vi "Spectrometer.vi"(0 "Function":T14, 3 "Labram HR Notifications":T13, 5 "Laser Settings":T5={"Laser Wavelength"=enum."633 nm", "Neutral Density Filter"=enum."1%"}, 7 "Spectrometer Settings":T2={"Confocal Hole Size (µm)"=150.0, "Grating"=1, "Detector"=enum."InGaAs Array"} {"Grating" items=["1800 l/mm", "150 l/mm"]}, 9 "Acquisition Settings":T1={"Acquisition Mode"=enum."Single Window", "Spectal Position (nm)"=480.0, "From (nm)"=632.0, "To (nm)"=1000.0, "Integration Time (s)"=3.0, "Number of Accumulations"=3, "AutoScanning"=FALSE, "Spike Removal"=FALSE}, 11 "error in":errorcluster, 12 "Optical Spectrum":enum32{"Energy", "Wavelength", "Raman Shift"}(tab), 13 "Path":path, 14 "LabramHR References":T8) -> (4 "Spectrum":T10, 6 "Laser Settings Out":T5={"Laser Wavelength"=enum."633 nm", "Neutral Density Filter"=enum."1%"}, 8 "Spectrometer Settings Out":T2={"Confocal Hole Size (µm)"=150.0, "Grating"=1, "Detector"=enum."InGaAs Array"} {"Grating" items=["1800 l/mm", "150 l/mm"]}, 10 "Acquisition Settings Out":T1={"Acquisition Mode"=enum."Single Window", "Spectal Position (nm)"=480.0, "From (nm)"=632.0, "To (nm)"=1000.0, "Integration Time (s)"=3.0, "Number of Accumulations"=3, "AutoScanning"=FALSE, "Spike Removal"=FALSE}, 15 "error out":errorcluster)   [LabVIEW 2014]
uses:
  Spectrometer Function.ctl
  Spectrometer Notifiers.ctl
  support/Instrument Status.ctl
  Laser Settings.ctl
  Laser.ctl
  Filter.ctl
  Grating Detector Settings.ctl
  Grating.ctl
  Detector.ctl
  Acquisition Settings.ctl
  Spectral Data.ctl
  Spectrometer Refnum.ctl
  Measurements/Plot Data/Optical Spectrum Plot Refnum.ctl
  MoveMotor Motor Name.ctl
  support/Instrument Status State.ctl
  Spectrometer Config.ctl
  Acquire Mode.ctl
  Acquire Shutter Mode.ctl
  Acquire Data Handling.ctl
panel:
  out "Detector Temperature":dbl
  out "Optical Spectrum vs Energy":cluster{"data":dbl[], "data":dbl[]}(graph)
  out "Optical Spectrum vs Wavelength":cluster{"data":dbl[], "data":dbl[]}(graph)
  out "Optical Spectrum vs Raman Shift":cluster{"data":dbl[], "data":dbl[]}(graph)
  out "Motor ID":T11={"Laser"=-1, "Hole"=-1, "Filter"=-1, "Grating"=-1, "Spectro"=-1, "Detector"=-1}
  out "Instrument Status":T12
  # "LICENSED MATERIALS – PROPERTY OF IBM\nCopyright IBM Corp. 2016,\nALL RIGHTS RESERVED"
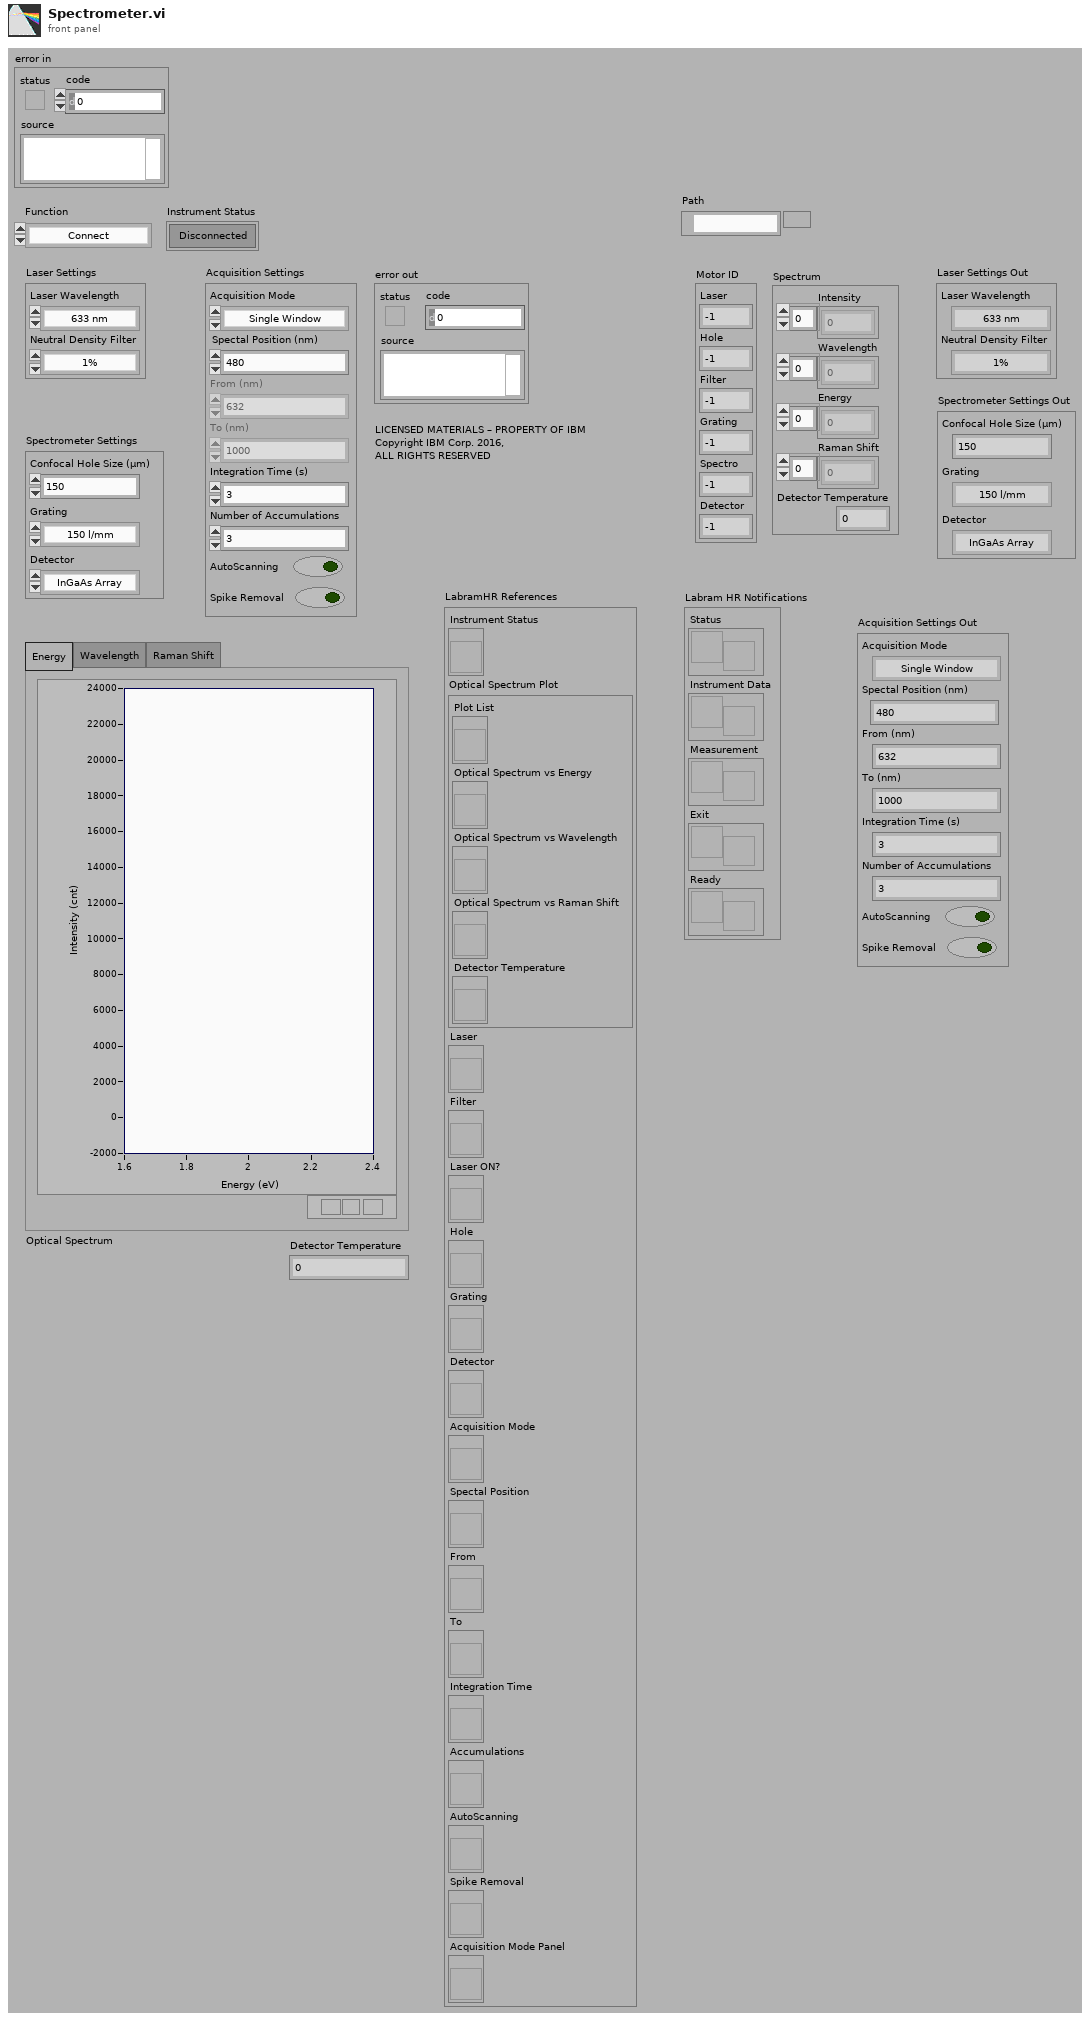
[diagram p1: front panel]
types:
  T1 = typedef "Acquisition Settings.ctl" = cluster{"Acquisition Mode":enum16{"Single Window", "Multi-Window"}, "Spectal Position (nm)":dbl, "From (nm)":dbl, "To (nm)":dbl, "Integration Time (s)":dbl, "Number of Accumulations":i32, "AutoScanning":bool, "Spike Removal":bool}
  T2 = typedef "Grating Detector Settings.ctl" = cluster{"Confocal Hole Size (µm)":dbl, "Grating":T3, "Detector":T4}
  T3 = typedef "Grating.ctl" = u16
  T4 = typedef "Detector.ctl" = enum16{"InGaAs Array", "Silicon CCD"}
  T5 = typedef "Laser Settings.ctl" = cluster{"Laser Wavelength":T6, "Neutral Density Filter":T7}
  T6 = typedef "Laser.ctl" = enum16{"633 nm", "784 nm", "532 nm", "365 nm"}
  T7 = typedef "Filter.ctl" = enum16{"100%", "50%", "25%", "10%", "1%", "0.1%", "0.01%"}
  T8 = typedef "Spectrometer Refnum.ctl" = cluster{"Instrument Status":refnum<vi>, "Optical Spectrum Plot":T9, "Laser":refnum<vi>, "Filter":refnum<vi>, "Laser ON?":refnum<vi>, "Hole":refnum<vi>, "Grating":refnum<vi>, "Detector":refnum<vi>, "Acquisition Mode":refnum<vi>, "Spectal Position":refnum<vi>, "From":refnum<vi>, "To":refnum<vi>, "Integration Time":refnum<vi>, "Accumulations":refnum<vi>, "AutoScanning":refnum<vi>, "Spike Removal":refnum<vi>, "Acquisition Mode Panel":refnum<vi>}
  T9 = typedef "Optical Spectrum Plot Refnum.ctl" = cluster{"Plot List":refnum<vi>, "Optical Spectrum vs Energy":refnum<vi>, "Optical Spectrum vs Wavelength":refnum<vi>, "Optical Spectrum vs Raman Shift":refnum<vi>, "Detector Temperature":refnum<vi>}
  T10 = typedef "Spectral Data.ctl" = cluster{"Intensity":dbl[], "Wavelength":dbl[], "Energy":dbl[], "Raman Shift":dbl[], "Detector Temperature":dbl}
  T11 = cluster{"Laser":i32, "Hole":i32, "Filter":i32, "Grating":i32, "Spectro":i32, "Detector":i32}
  T12 = typedef "Instrument Status.ctl" = bool
  T13 = typedef "Spectrometer Notifiers.ctl" = cluster{"Status":refnum<notifier>, "Instrument Data":refnum<notifier>, "Measurement":refnum<notifier>, "Exit":refnum<notifier>, "Ready":refnum<notifier>}
  T14 = typedef "Spectrometer Function.ctl" = enum16{"Connect", "Complete Configuration", "Get Status", "Load Configuration", "Save Configuration", "Acquire Spectrum", "Read File", "Set Laser", "Set Filter", "Set Hole", "Set Grating", "Set Grating Position", "Set Detector", "Set Acquisition Mode", "Update Refnums", "Disconnect"}
  T15 = enum16{"Generic Data", "Spectrum", "Spectral Profile Image", "Map", "Video", "First Data", "Next Data"}
  T16 = typedef "Instrument Status State.ctl" = enum16{"Unknown", "Idle", "Standby", "Configuring", "Measuring", "Moving", "Disconnected"}
  T17 = typedef "MoveMotor Motor Name.ctl" = enum16{"Spectro", "Premono", "Grating", "Slit", "Hole", "X", "Y", "XT", "YT", "XL", "YL", "Z", "Laser", "Filter", "Objective", "Detector", "Detector Temperature"}
  T18 = typedef "Spectrometer Config.ctl" = cluster{"Laser Settings":T5, "Spectrometer Settings":T2, "Acquisition Settings":T1, "Path":path}
  T19 = enum8{"Enabled", "Disabled", "Disabled and Grayed Out"}
  T20 = cluster{"Optical Spectrum vs Energy":cluster{"Intensity":dbl[], "Energy":dbl[]}, "Optical Spectrum vs Wavelength":cluster{"Intensity":dbl[], "Wavelength":dbl[]}, "Optical Spectrum vs Raman Shift":cluster{"Intensity":dbl[], "Raman Shift":dbl[]}}
  T21 = typedef "Acquire Mode.ctl" = u16
  T22 = typedef "Acquire Shutter Mode.ctl" = u16
  T23 = typedef "Acquire Data Handling.ctl" = u16
  T24 = enum8{"Enabled", "Disabled", "Disabled and Grayed Out"}[]
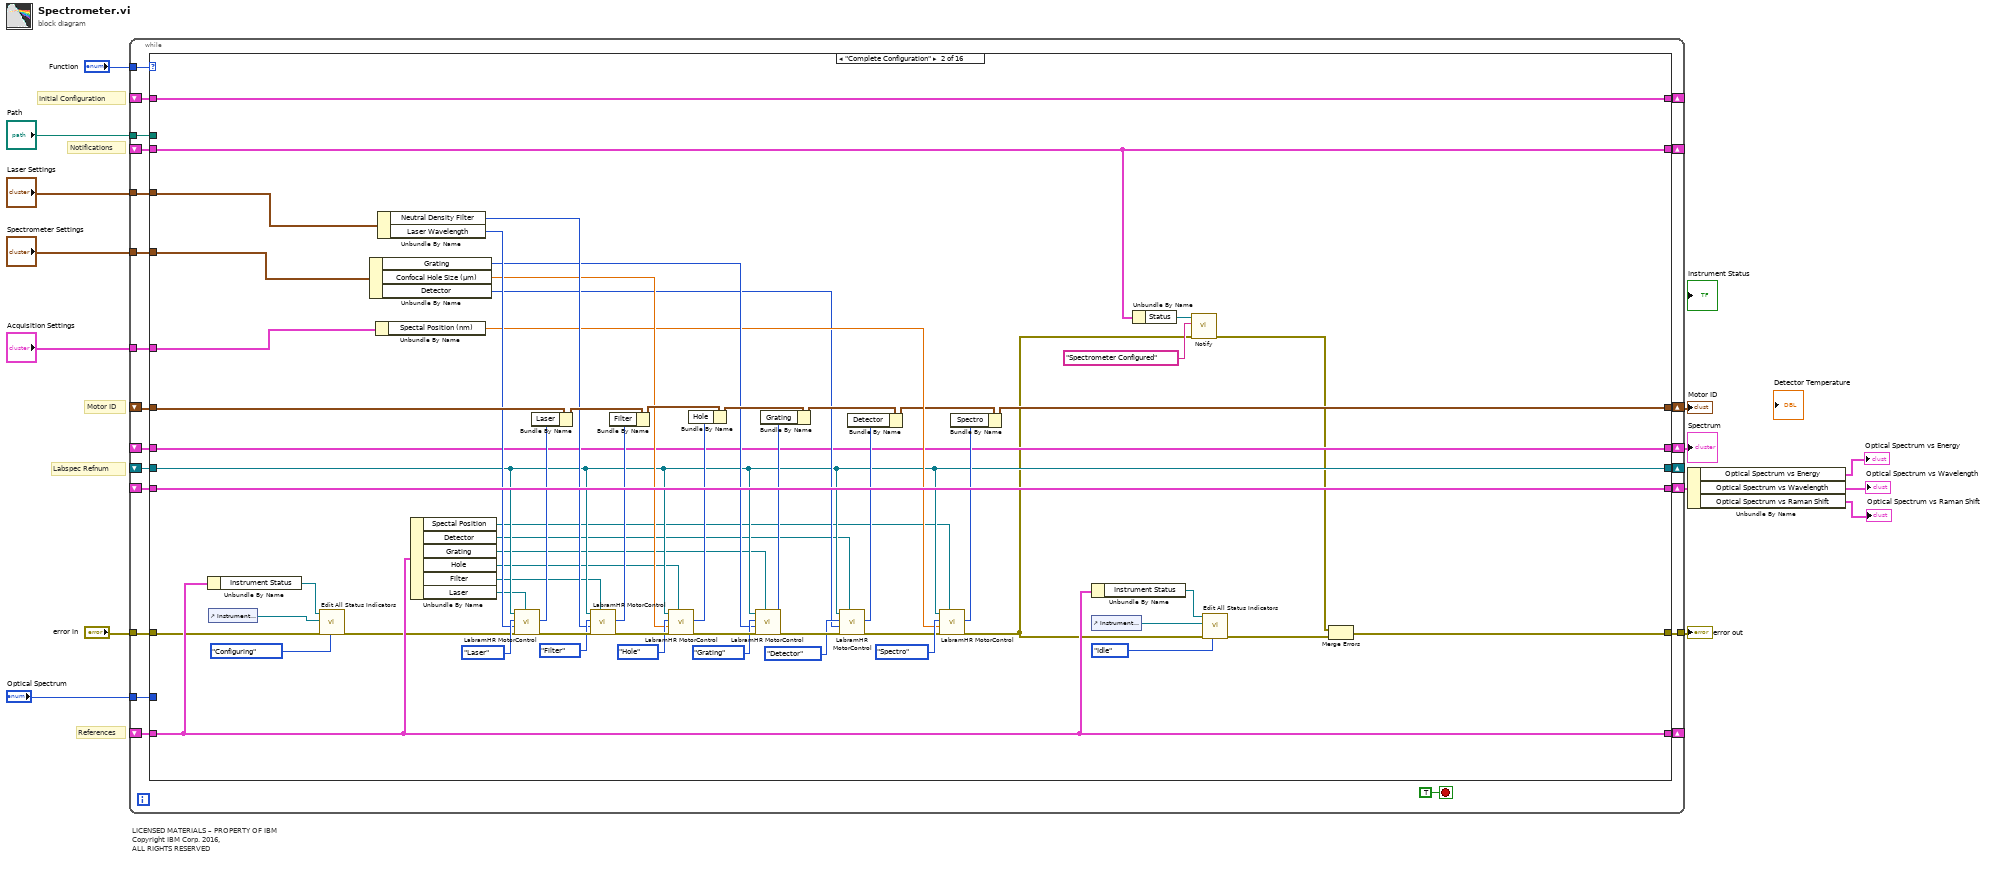
[diagram p0: block diagram]
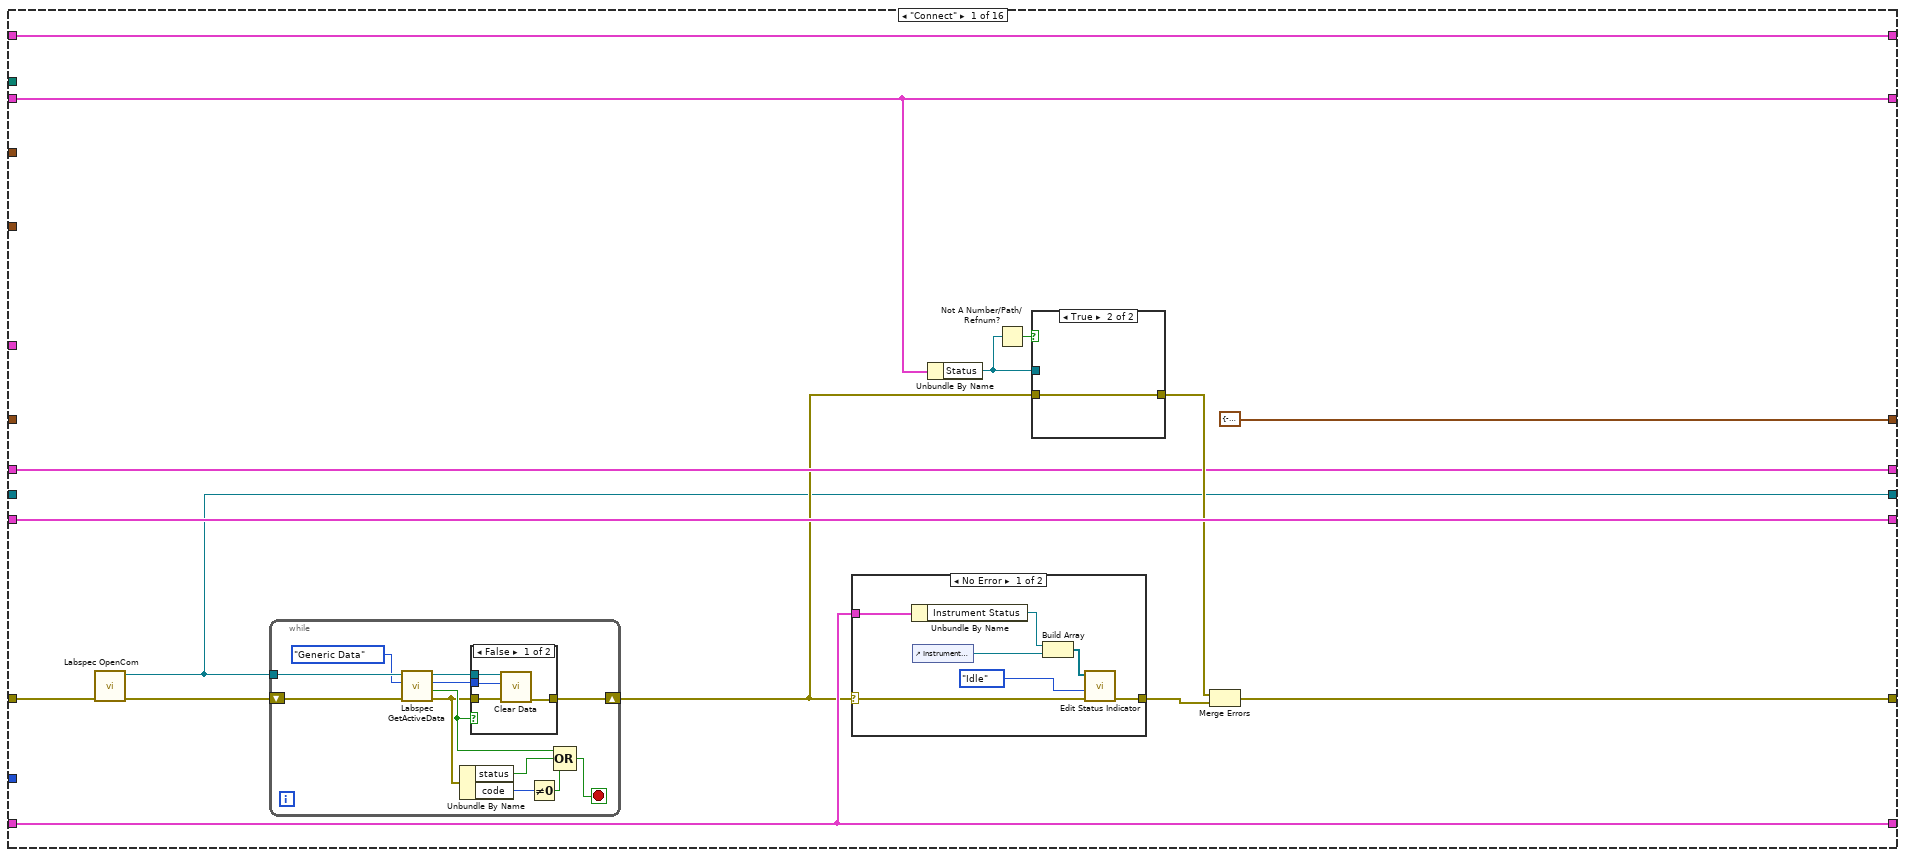
[diagram p2: hidden frame]
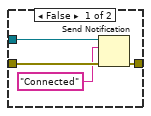
[diagram p4: hidden frame]
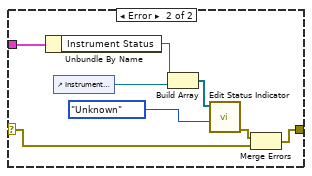
[diagram p5: hidden frame]
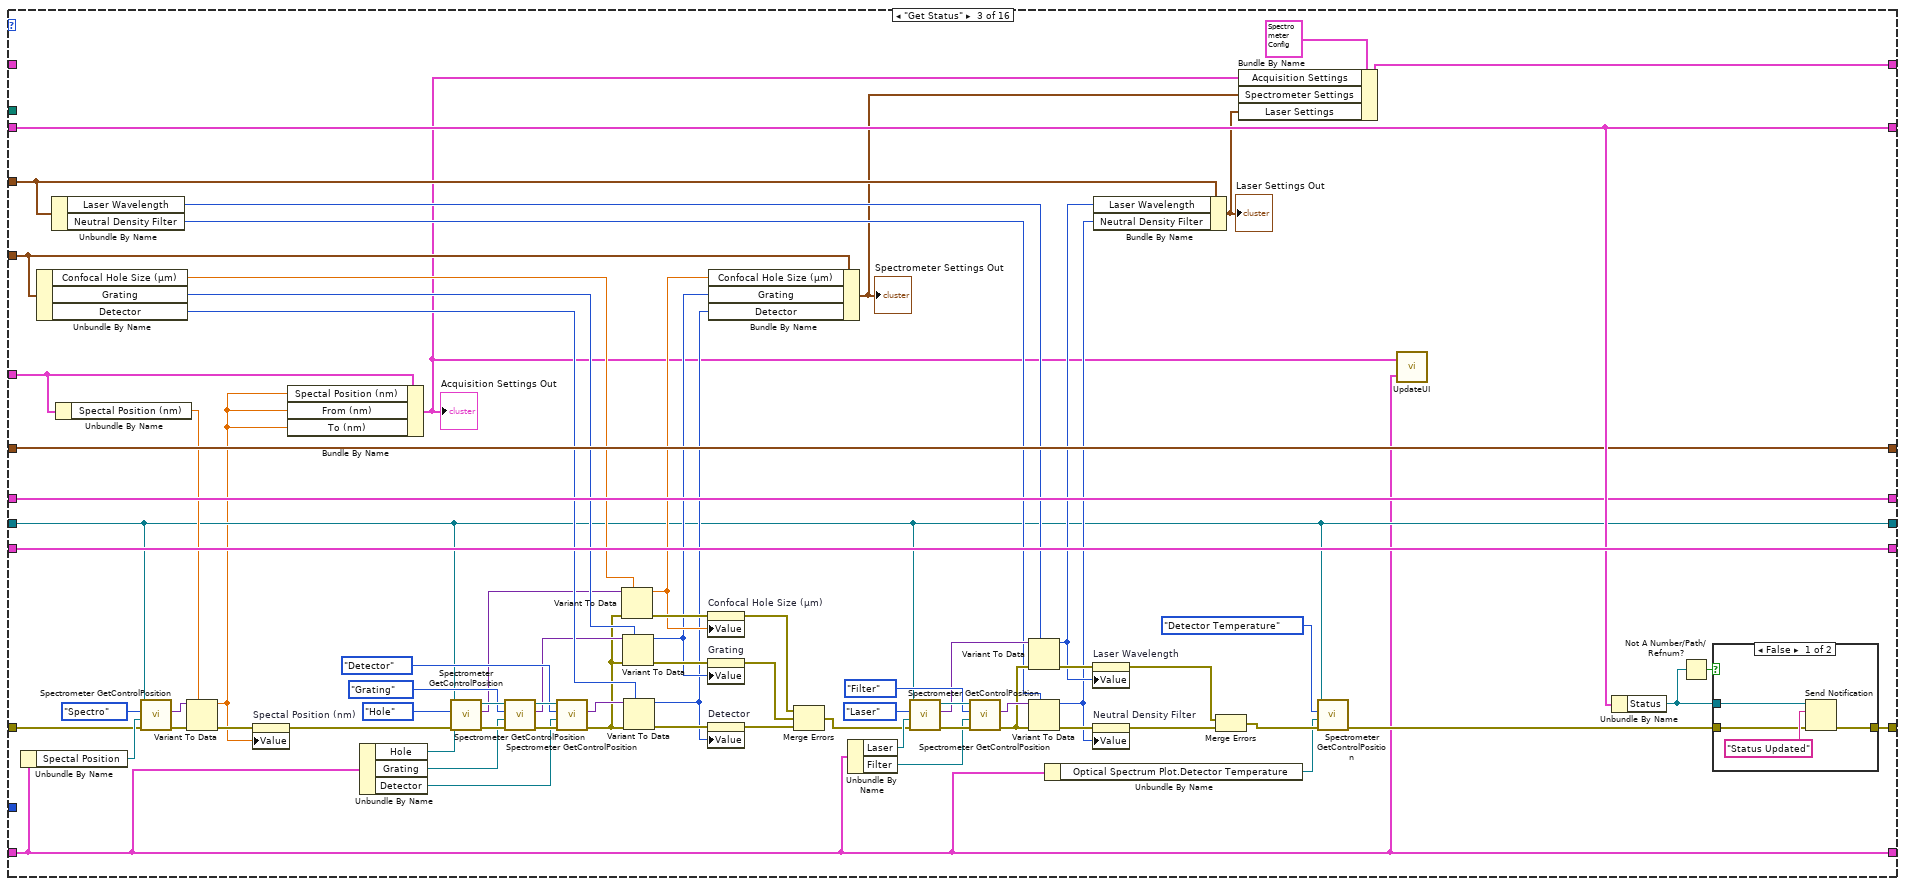
[diagram p6: hidden frame]
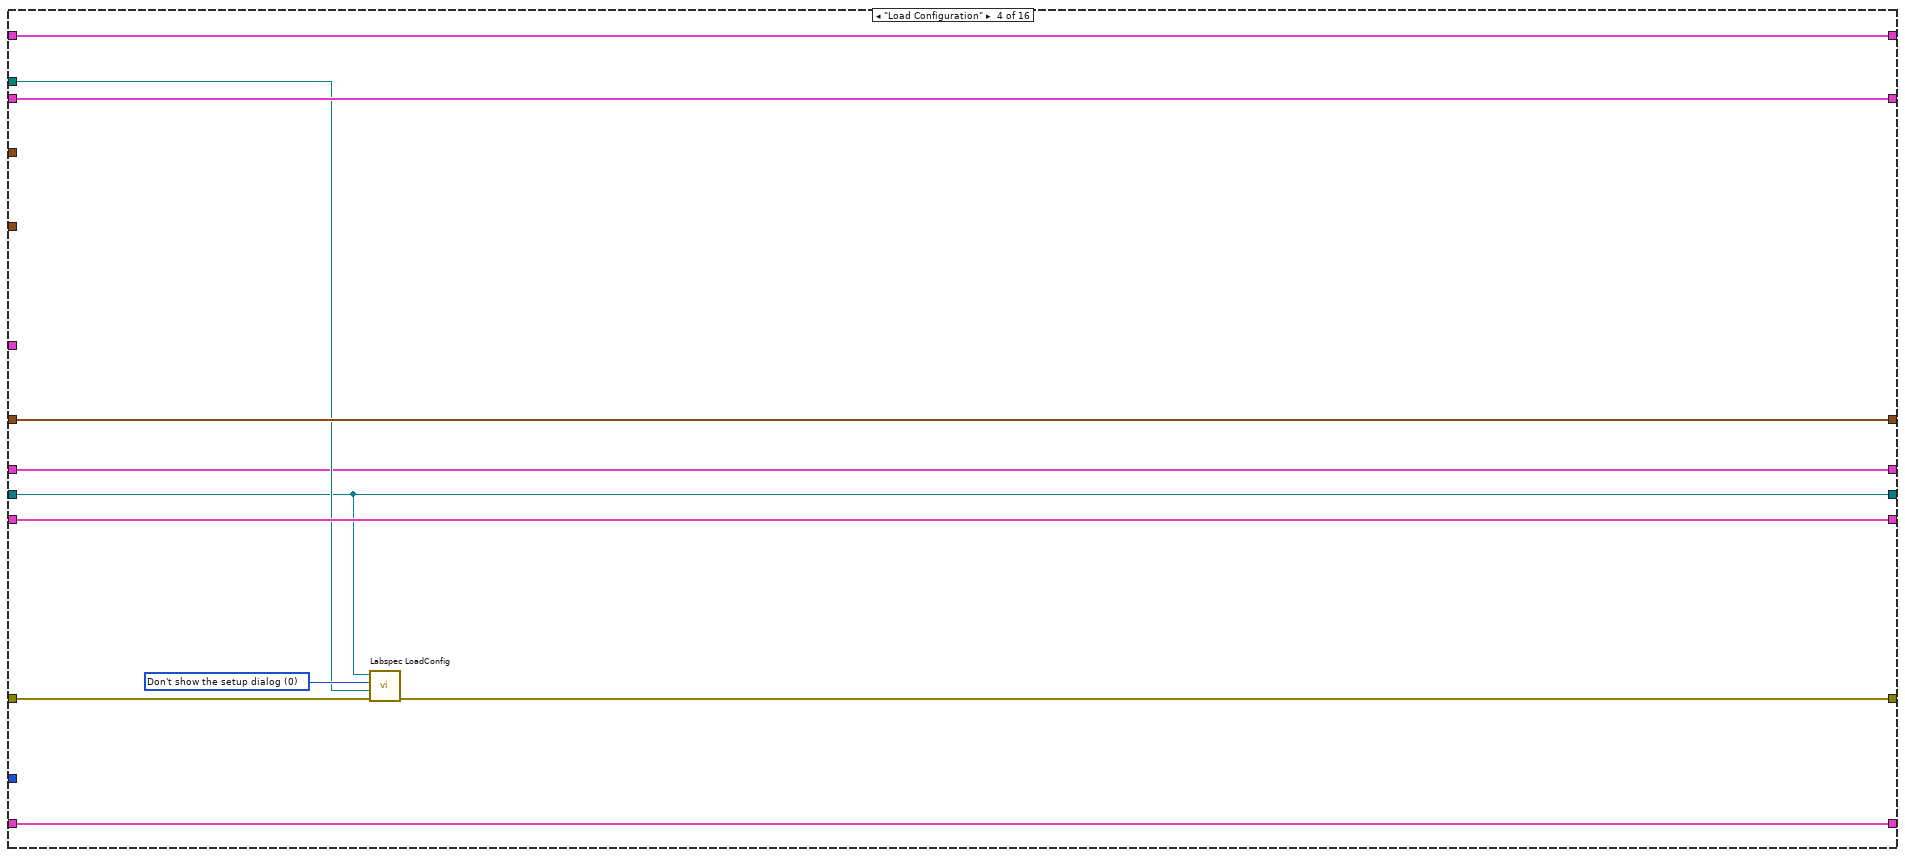
[diagram p8: hidden frame]
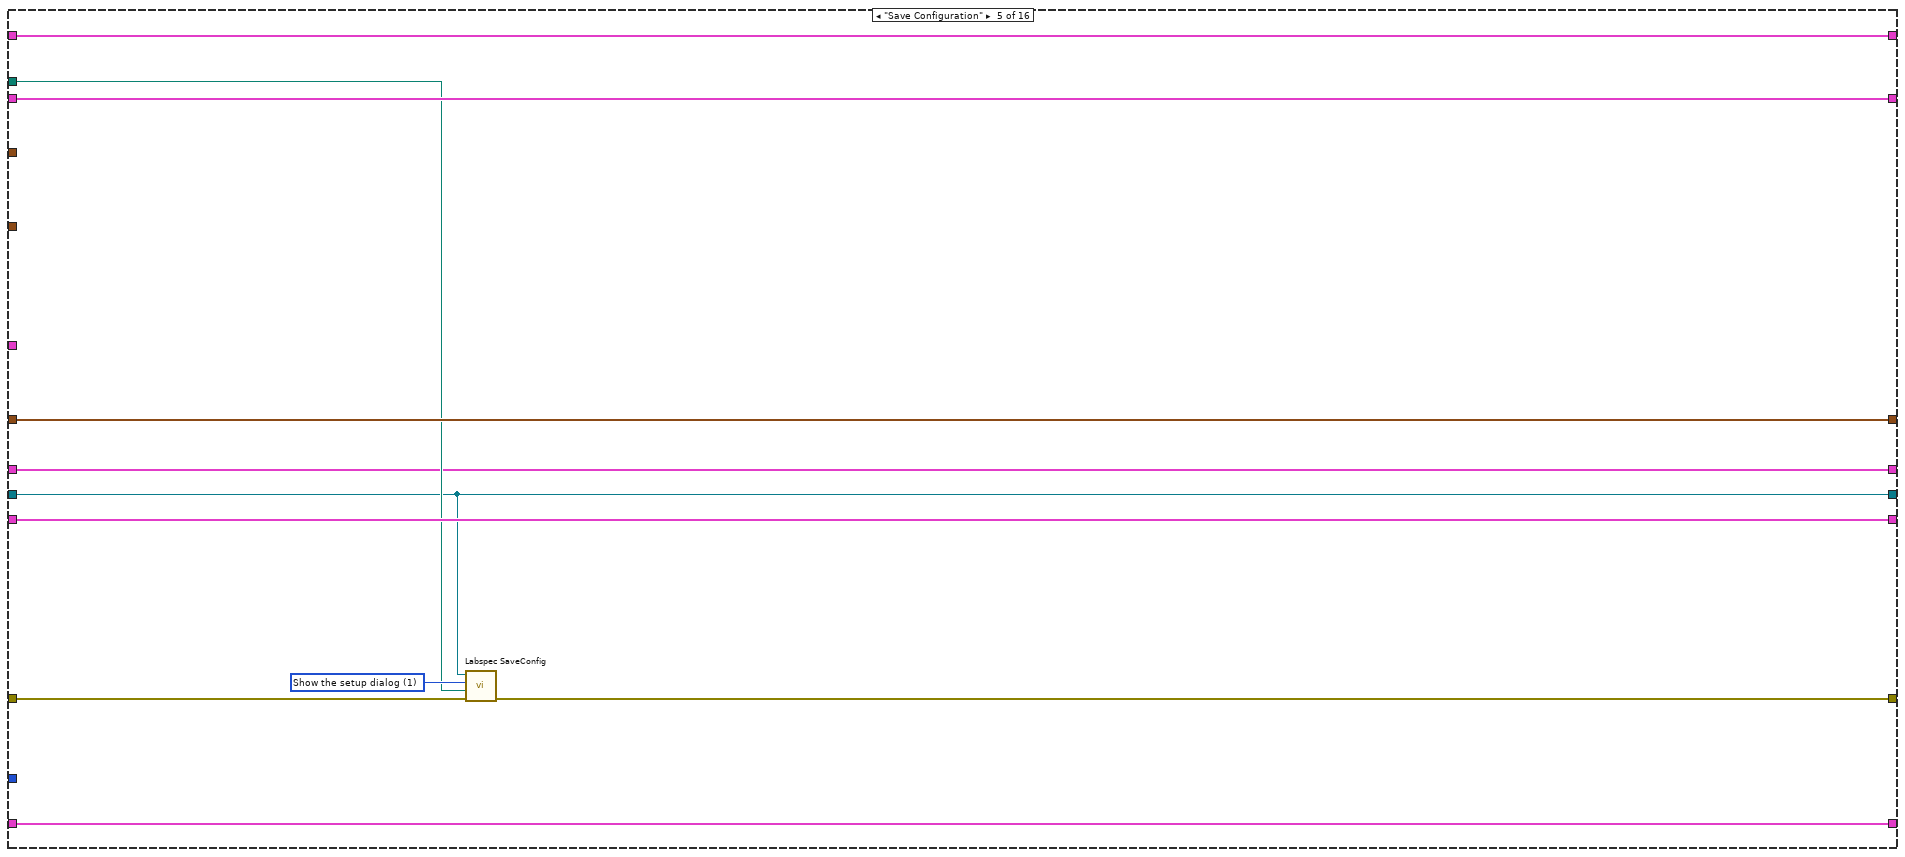
[diagram p9: hidden frame]
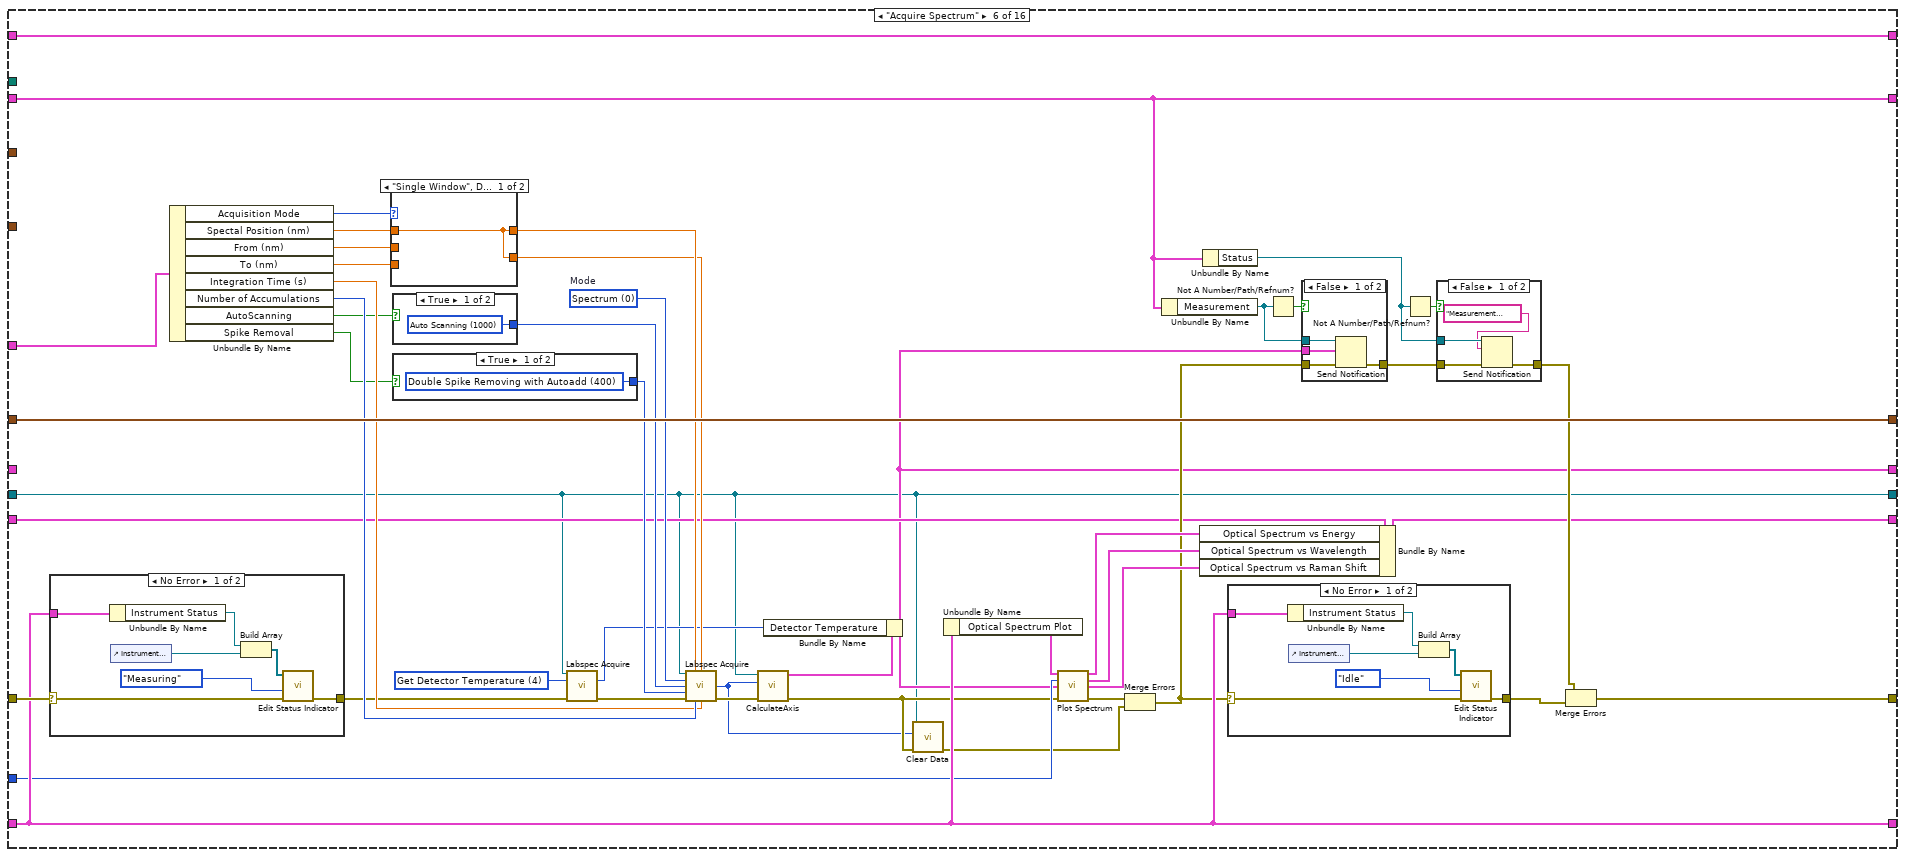
[diagram p10: hidden frame]
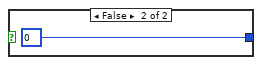
[diagram p13: hidden frame]
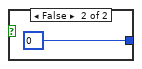
[diagram p14: hidden frame]
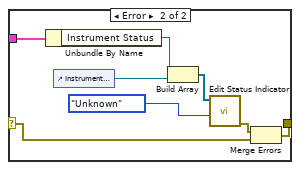
[diagram p15: hidden frame]
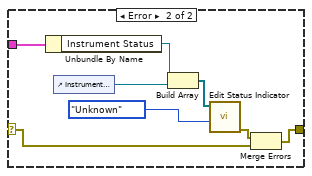
[diagram p16: hidden frame]
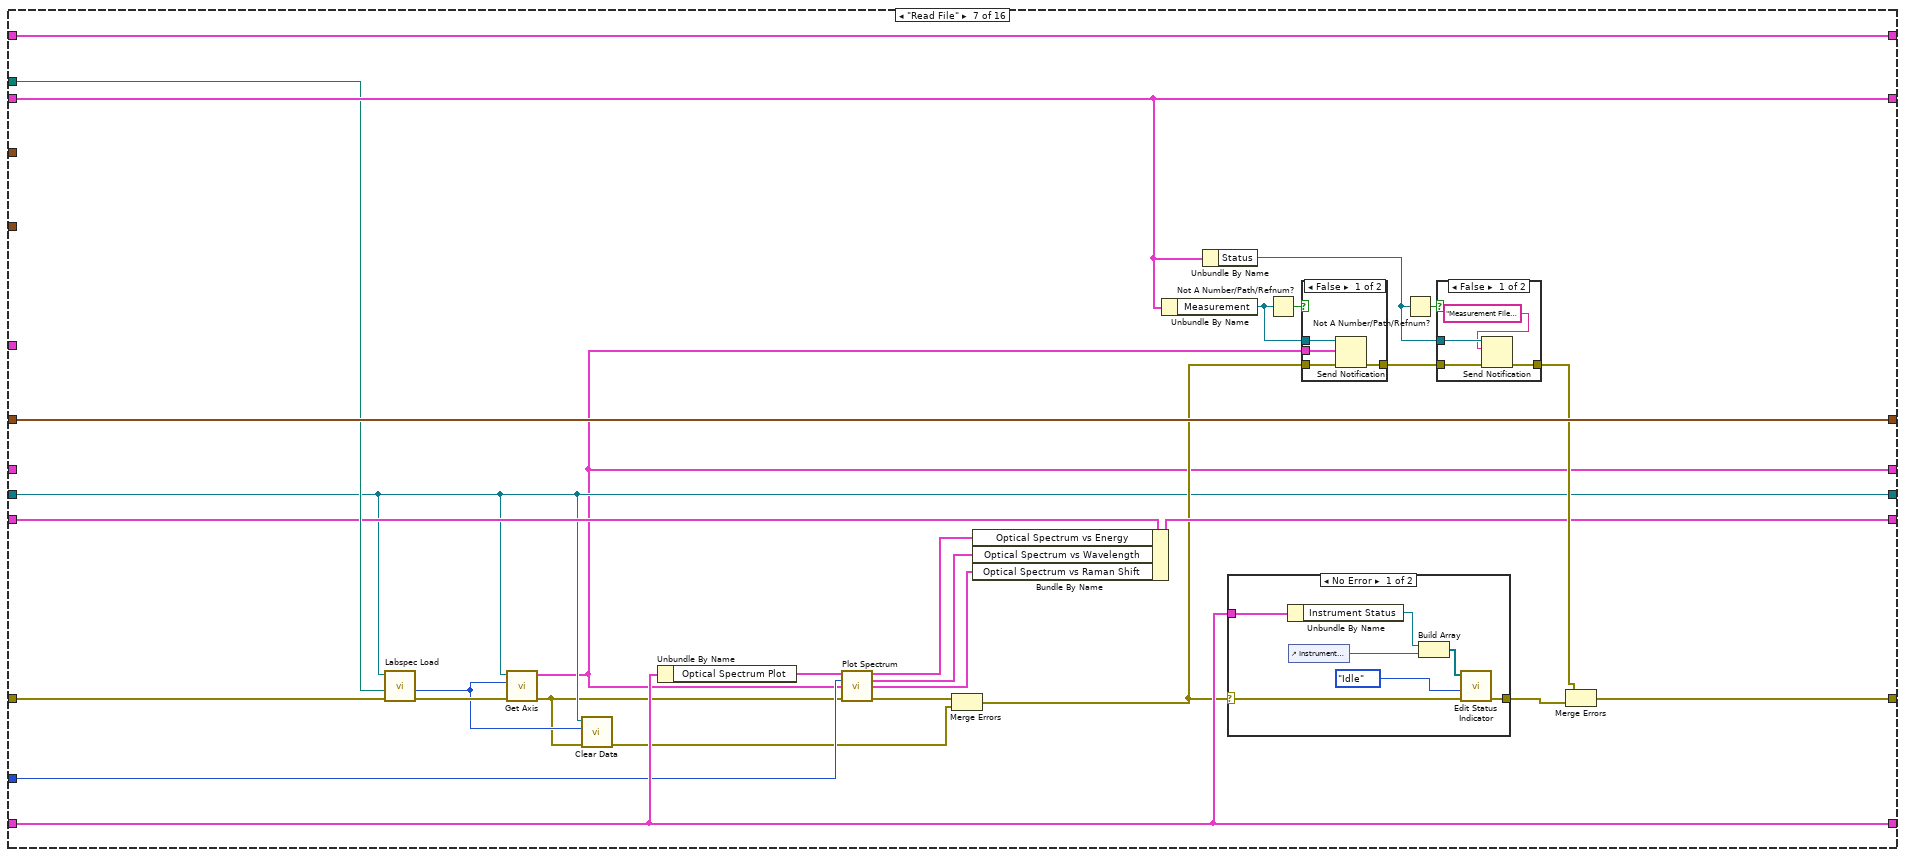
[diagram p18: hidden frame]
diagram:
  # "LICENSED MATERIALS – PROPERTY OF IBM\nCopyright IBM Corp. 2016,\nALL RIGHTS RESERVED"
  # "Initial Configuration"
  # "Notifications"
  # "References"
  # "Motor ID"
  # "Labspec Refnum"
  n1 = while {
    tunnel: "Function" -> [w37]
    tunnel: "error in" -> [w35]
    tunnel: [w34] -> w13
    shift-right: [w33] -> _
    shift-left: _ -> [w32]
    shift-right: [w31] -> w5
    shift-left: _ -> [w30]
    shift-right: [w29] -> w7
    shift-left: _ -> [w28]
    shift-right: [w27] -> _
    shift-left: _ -> [w26]
    shift-right: [w25] -> _
    shift-left: _ -> [w24]
    tunnel: "Laser Settings" -> [w23]
    tunnel: "Spectrometer Settings" -> [w22]
    tunnel: "Acquisition Settings" -> [w21]
    tunnel: "Path" -> [w20]
    shift-right: [w19] -> w6
    shift-left: _ -> [w18]
    tunnel: "Optical Spectrum" -> [w17]
    shift-right: [w16] -> _
    shift-left: _ -> [w15]
    stop <- TRUE stop-if-true
    n2 = case shown="\"Complete Configuration\"" w37 {
      tunnel: w35 -> [w52 w91 w198 w238 w249 w295 w360 w414 w470 w525 w591 w647 w710 w774 w805 w827]
      tunnel: [w44 w113 w190 w237 w248 w271 w362 w404 w462 w517 w586 w640 w703 w758 w804 w862] -> w34
      tunnel: [w39 w109 w161 w230 w241 w251 w347 w410 w466 w521 w576 w642 w695 w777 w811 w824] -> w33
      tunnel: w32 -> [_ w109 w161 w230 w241 w251 w347 w410 w466 w521 w576 w642 w695 w777 w811 w824]
      tunnel: [w42 w111 w217 w229 w240 w253 w346 w409 w465 w520 w587 w641 w697 w779 w803 w859] -> w19
      tunnel: [w51 w148 w222 w235 w246 w269 w358 w418 w471 w527 w592 w648 w711 w775 T20 {"Optical Spectrum vs Energy"={"Intensity"=[], "Energy"=[]}, "Optical Spectrum vs Wavelength"={"Intensity"=[], "Wavelength"=[]}, "Optical Spectrum vs Raman Shift"={"Intensity"=[], "Raman Shift"=[]}} w867] -> w31
      tunnel: w30 -> [w51 w148 w222 w235 w246 w254 w357 w418 w471 w527 w592 w648 w711 w775 _ w867]
      tunnel: [T11 {"Laser"=-1, "Hole"=-1, "Filter"=-1, "Grating"=-1, "Spectro"=-1, "Detector"=-1} ("Motor ID 2") w135 w216 w234 w245 w296 w372 w415 w472 w528 w593 w649 w712 w776 w810 w828] -> w29
      tunnel: w28 -> [_ w145 w216 w234 w245 w296 w372 w416 w473 w529 w594 w650 w713 w776 w810 w829]
      tunnel: [w49 w108 w151 w233 w244 w278 w369 w399 w456 w526 w577 w644 w692 w757 "LabramHR References" w823] -> w27
      tunnel: w26 -> [w49 w108 w151 w233 w244 w278 w369 w399 w456 w526 w577 w644 w692 w757 _ w823]
      tunnel: [w45 w112 w218 w232 w243 w272 w363 w406 w459 w514 w582 w635 w700 w778 "Labram HR Notifications" w864] -> w25
      tunnel: w24 -> [w45 w112 w218 w232 w243 w272 w363 w406 w459 w514 w582 w635 w700 w778 _ w864]
      tunnel: w23 -> [_ w127 w169 _ _ _ _ w402 w458 _ _ _ _ _ _ _]
      tunnel: w22 -> [_ w124 w166 _ _ _ _ _ _ w512 w581 _ w706 _ _ _]
      tunnel: w21 -> [_ w121 w152 _ _ w293 _ _ _ _ w571 w633 _ w764 _ _]
      tunnel: w20 -> [_ _ _ w231 w242 _ w359 _ _ _ _ _ _ _ _ _]
      tunnel: w18 -> [w42 w111 w217 w229 w240 _ _ w409 w465 w520 w587 w641 w704 w779 w803 w859]
      tunnel: w17 -> [_ _ _ _ _ w265 w353 _ _ _ _ _ _ _ _ _]
      tunnel: [w38 w110 w155 w228 w239 w250 w344 w398 w454 w510 w566 w631 w687 w761 w801 w830] -> w16
      tunnel: w15 -> [w38 w110 _ w228 w239 w250 w344 w398 w454 w510 w566 w631 w687 w761 w801 w830]
      frame "Connect" {
        n3 = call "Labspec OpenCom.vi"("error in"=w52) -> ("error out"=w41:errorcluster, "Automation Refnum"=w39:refnum<k7>)  [unwired: 9 out]
        n4 = while {
          shift-right: [w61] -> w40
          shift-left: w41 -> [w62]
          tunnel: w39 -> [w63]
          stop <- w54 stop-if-true
          n5 = call "Labspec GetActiveData.vi"("error in"=w62, "Data Type"=T15."Generic Data", "Automation Refnum In"=w63) -> ("error out"=w58:errorcluster, "No Active Data?"=w59:bool, "Data ID"=w53:i32, "Automation Refnum Out"=w64:refnum<k7>)  [unwired: 5 in]
          n6 = Unbundle By Name(w58) -> ("status"=w57:bool, "code"=w56:i32)
          n7 = case shown="False" w59 {
            tunnel: w64 -> [w68 _]
            tunnel: w58 -> [w67 w69]
            tunnel: [w66 w69] -> w61
            tunnel: w53 -> [w65 _]
            frame False {
              n8 = call "Clear Data.vi"("error in (no error)"=w67, "AcqID"=w65, "Automation Refnum in"=w68) -> ("error out"=w66:errorcluster)  [unwired: 8 in]
            }
            frame True {
            }
          }
          n9 = Not Equal To 0?(x=w56) -> (x != 0?=w55:bool)
          n10 = Compound Arithmetic op=OR(w59, w57, w55) -> (w54:bool)
        }
        n11 = case shown="No Error" w40 {
          selector: w40 -> [w80 w84]
          tunnel: [w79 w83] -> w48
          tunnel: w49 -> [w75 w85]
          frame No Error {
            n12 = Unbundle By Name(w75) -> ("Instrument Status"=w76:refnum<vi>)
            n13 = control-ref of="Instrument Status"() -> (w78:refnum<vi>)
            n14 = Build Array(w76, w78) -> (w77:refnum<vi>[])
            n15 = call "Edit Status Indicator.vi"("error in (no error)"=w80, "State"=Instrument_Status_State."Idle", "Instrument Status Refnum"=w77) -> ("error out"=w79:errorcluster)  [unwired: 1 in, 7 out]
          }
          frame Error {
            n16 = Unbundle By Name(w85) -> ("Instrument Status"=w86:refnum<vi>)
            n17 = control-ref of="Instrument Status"() -> (w88:refnum<vi>)
            n18 = Build Array(w86, w88) -> (w87:refnum<vi>[])
            n19 = call "Edit Status Indicator.vi"("State"=Instrument_Status_State."Unknown", "Instrument Status Refnum"=w87) -> ("error out"=w82:errorcluster)  [unwired: 2 in, 7 out]
            n20 = Merge Errors(w82, w84) -> (w83:errorcluster)
          }
        }
        n21 = Unbundle By Name(w45) -> ("Status"=w47:refnum<notifier>)
        n22 = Not A Number/Path/Refnum?(number/path/refnum=w47) -> (NaN/Path/Refnum?=w46:bool)
        n23 = case shown="True" w46 {
          tunnel: w40 -> [w73 w74]
          tunnel: [w72 w74] -> w43
          tunnel: w47 -> [w71 _]
          frame False {
            n24 = Send Notification(notification="Connected", notifier=w71, error in (no error)=w73) -> (error out=w72:errorcluster)  [unwired: 1 out]
          }
          frame True {
          }
        }
        n25 = Merge Errors(w43, w48) -> (w44:errorcluster)
      }
      frame "Complete Configuration" {
        n26 = Unbundle By Name(w108) -> ("Instrument Status"=w94:refnum<vi>)
        n27 = control-ref of="Instrument Status"() -> (w93:refnum<vi>)
        n28 = call "Edit All Status Indicators.vi"("Instrument Status Ouside"=w94, "Instrument Status Inside"=w93, "Error In"=w91, "State"=Instrument_Status_State."Configuring") -> ("Error Out"=w90:errorcluster)  [unwired: 6 in]
        n29 = Unbundle By Name(w124) -> ("Grating"=w122:T3, "Confocal Hole Size (µm)"=w123:dbl, "Detector"=w114:T4)
        n30 = Unbundle By Name(w121) -> ("Spectal Position (nm)"=w120:dbl)
        n31 = Unbundle By Name(w127) -> ("Neutral Density Filter"=w125:T7, "Laser Wavelength"=w126:T6)
        n32 = Unbundle By Name(w108) -> ("Spectal Position"=w102:refnum<vi>, "Detector"=w103:refnum<vi>, "Grating"=w104:refnum<vi>, "Hole"=w105:refnum<vi>, "Filter"=w106:refnum<vi>, "Laser"=w107:refnum<vi>)
        n33 = call "LabramHR MotorControl.vi"("Control Refnum"=w107, "error in"=w90, "Destination"=w126, "Motor Name"=MoveMotor_Motor_Name."Laser", "Automation Refnum In"=w109) -> ("error out"=w146:errorcluster, "MotorID"=w134:i32)  [unwired: 1 in, 4 out]
        n34 = Bundle By Name(cluster=w145, "Laser"=w134) -> (w144:T11)
        n35 = call "LabramHR MotorControl.vi"("Control Refnum"=w106, "error in"=w146, "Destination"=w125, "Motor Name"=MoveMotor_Motor_Name."Filter", "Automation Refnum In"=w109) -> ("error out"=w143:errorcluster, "MotorID"=w147:i32)  [unwired: 1 in, 4 out]
        n36 = Bundle By Name(cluster=w144, "Filter"=w147) -> (w138:T11)
        n37 = call "LabramHR MotorControl.vi"("Control Refnum"=w105, "error in"=w143, "Destination"=w123, "Motor Name"=MoveMotor_Motor_Name."Hole", "Automation Refnum In"=w109) -> ("error out"=w141:errorcluster, "MotorID"=w142:i32)  [unwired: 1 in, 4 out]
        n38 = Bundle By Name(cluster=w138, "Hole"=w142) -> (w137:T11)
        n39 = call "LabramHR MotorControl.vi"("Control Refnum"=w104, "error in"=w141, "Destination"=w122, "Motor Name"=MoveMotor_Motor_Name."Grating", "Automation Refnum In"=w109) -> ("error out"=w119:errorcluster, "MotorID"=w139:i32)  [unwired: 1 in, 4 out]
        n40 = Bundle By Name(cluster=w137, "Grating"=w139) -> (w136:T11)
        n41 = call "LabramHR MotorControl.vi"("Control Refnum"=w103, "error in"=w119, "Destination"=w114, "Motor Name"=MoveMotor_Motor_Name."Detector", "Automation Refnum In"=w109) -> ("error out"=w118:errorcluster, "MotorID"=w116:i32)  [unwired: 1 in, 4 out]
        n42 = Bundle By Name(cluster=w136, "Detector"=w116) -> (w117:T11)
        n43 = call "LabramHR MotorControl.vi"("Control Refnum"=w102, "error in"=w118, "Destination"=w120, "Motor Name"=MoveMotor_Motor_Name."Spectro", "Automation Refnum In"=w109) -> ("error out"=w99:errorcluster, "MotorID"=w140:i32)  [unwired: 1 in, 4 out]
        n44 = Bundle By Name(cluster=w117, "Spectro"=w140) -> (w135:T11)
        n45 = Unbundle By Name(w108) -> ("Instrument Status"=w97:refnum<vi>)
        n46 = control-ref of="Instrument Status"() -> (w96:refnum<vi>)
        n47 = Unbundle By Name(w112) -> ("Status"=w101:refnum<notifier>)
        n48 = call "Notify.vi"("error in (no error)"=w99, "String"="Spectrometer Configured", "Notifier in"=w101) -> ("error out"=w98:errorcluster)  [unwired: 8 in]
        n49 = call "Edit All Status Indicators.vi"("Instrument Status Ouside"=w97, "Instrument Status Inside"=w96, "Error In"=w99, "State"=Instrument_Status_State."Idle") -> ("Error Out"=w133:errorcluster)  [unwired: 6 in]
        n50 = Merge Errors(w98, w133) -> (w113:errorcluster)
      }
      frame "Get Status" {
        n51 = Unbundle By Name(w151) -> ("Spectal Position"=w199:refnum<vi>)
        n52 = Unbundle By Name(w166) -> ("Confocal Hole Size (µm)"=w187:dbl, "Grating"=w188:T3, "Detector"=w189:T4)
        n53 = Unbundle By Name(w169) -> ("Laser Wavelength"=w175:T6, "Neutral Density Filter"=w174:T7)
        n54 = Unbundle By Name(w152) -> ("Spectal Position (nm)"=w197:dbl)
        n55 = call "Spectrometer GetControlPosition.vi"("error in"=w198, "Control Refnum"=w199, "Motor Name"=MoveMotor_Motor_Name."Spectro", "Automation Refnum In"=w161) -> ("error out"=w195:errorcluster, "Position"=w196:variant)  [unwired: 5 in, 1 out]
        n56 = Variant To Data(error in=w195, type=w197, Variant=w196) -> (data=w149:dbl, error out=w194:errorcluster)
        n57 = property on="Spectal Position (nm)" class="DigNum (strict)"(error in=w194, "Value"=w149) -> (error out=w162:errorcluster)  [unwired: 1 in, 1 out]
        n58 = Bundle By Name(cluster=w152, "Spectal Position (nm)"=w149, "From (nm)"=w149, "To (nm)"=w149) -> (w150:T1)
        "Acquisition Settings Out" <- w150
        n59 = Unbundle By Name(w151) -> ("Hole"=w200:refnum<vi>, "Grating"=w202:refnum<vi>, "Detector"=w201:refnum<vi>)
        n60 = call "Spectrometer GetControlPosition.vi"("error in"=w162, "Control Refnum"=w200, "Motor Name"=MoveMotor_Motor_Name."Hole", "Automation Refnum In"=w161) -> ("error out"=w211:errorcluster, "Position"=w184:variant, "Automation Refnum Out"=w214:refnum<k7>)  [unwired: 5 in]
        n61 = call "Spectrometer GetControlPosition.vi"("error in"=w211, "Control Refnum"=w202, "Motor Name"=MoveMotor_Motor_Name."Grating", "Automation Refnum In"=w214) -> ("error out"=w210:errorcluster, "Position"=w185:variant, "Automation Refnum Out"=w215:refnum<k7>)  [unwired: 5 in]
        n62 = call "Spectrometer GetControlPosition.vi"("error in"=w210, "Control Refnum"=w201, "Motor Name"=MoveMotor_Motor_Name."Detector", "Automation Refnum In"=w215) -> ("error out"=w183:errorcluster, "Position"=w186:variant)  [unwired: 5 in, 1 out]
        n63 = Variant To Data(error in=w183, type=w187, Variant=w184) -> (data=w165:dbl, error out=w182:errorcluster)
        n64 = Variant To Data(error in=w183, type=w188, Variant=w185) -> (data=w164:T3, error out=w181:errorcluster)
        n65 = Variant To Data(error in=w183, type=w189, Variant=w186) -> (data=w163:T4, error out=w180:errorcluster)
        n66 = property on="Confocal Hole Size (µm)" class="DigNum (strict)"(error in=w182, "Value"=w165) -> (error out=w179:errorcluster)  [unwired: 1 in, 1 out]
        n67 = property on="Grating" class="Ring (strict)"(error in=w181, "Value"=w164) -> (error out=w178:errorcluster)  [unwired: 1 in, 1 out]
        n68 = property on="Detector" class="Enum (strict)"(error in=w180, "Value"=w163) -> (error out=w177:errorcluster)  [unwired: 1 in, 1 out]
        n69 = Bundle By Name(cluster=w166, "Confocal Hole Size (µm)"=w165, "Grating"=w164, "Detector"=w163) -> (w153:T2)
        "Spectrometer Settings Out" <- w153
        n70 = Merge Errors(w179, w178, w177) -> (w176:errorcluster)
        n71 = Unbundle By Name(w151) -> ("Laser"=w204:refnum<vi>, "Filter"=w203:refnum<vi>)
        n72 = call "Spectrometer GetControlPosition.vi"("error in"=w176, "Control Refnum"=w204, "Motor Name"=MoveMotor_Motor_Name."Laser", "Automation Refnum In"=w161) -> ("error out"=w212:errorcluster, "Position"=w192:variant, "Automation Refnum Out"=w213:refnum<k7>)  [unwired: 5 in]
        n73 = call "Spectrometer GetControlPosition.vi"("error in"=w212, "Control Refnum"=w203, "Motor Name"=MoveMotor_Motor_Name."Filter", "Automation Refnum In"=w213) -> ("error out"=w191:errorcluster, "Position"=w193:variant)  [unwired: 5 in, 1 out]
        n74 = Variant To Data(error in=w191, type=w175, Variant=w192) -> (data=w168:T6, error out=w172:errorcluster)
        n75 = Variant To Data(error in=w191, type=w174, Variant=w193) -> (data=w167:T7, error out=w173:errorcluster)
        n76 = Unbundle By Name(w151) -> ("Optical Spectrum Plot.Detector Temperature"=w157:refnum<vi>)
        n77 = property on="Laser Wavelength" class="Enum (strict)"(error in=w172, "Value"=w168) -> (error out=w170:errorcluster)  [unwired: 1 in, 1 out]
        n78 = property on="Neutral Density Filter" class="Enum (strict)"(error in=w173, "Value"=w167) -> (error out=w171:errorcluster)  [unwired: 1 in, 1 out]
        n79 = Bundle By Name(cluster=w169, "Laser Wavelength"=w168, "Neutral Density Filter"=w167) -> (w154:T5)
        "Laser Settings Out" <- w154
        n80 = Merge Errors(w170, w171) -> (w159:errorcluster)
        n81 = Bundle By Name(cluster=T18 {"Laser Settings"={"Laser Wavelength"=enum."633 nm", "Neutral Density Filter"=enum."1%"}, "Spectrometer Settings"={"Confocal Hole Size (µm)"=150.0, "Grating"=1, "Detector"=enum."InGaAs Array"}, "Acquisition Settings"={"Acquisition Mode"=enum."Single Window", "Spectal Position (nm)"=480.0, "From (nm)"=632.0, "To (nm)"=1000.0, "Integration Time (s)"=3.0, "Number of Accumulations"=3, "AutoScanning"=FALSE, "Spike Removal"=FALSE}, "Path"=path ""} ("LabramHR"), "Acquisition Settings"=w150, "Spectrometer Settings"=w153, "Laser Settings"=w154) -> (w155:T18)
        n82 = call "Spectrometer GetControlPosition.vi"("error in"=w159, "Control Refnum"=w157, "Motor Name"=MoveMotor_Motor_Name."Detector Temperature", "Automation Refnum In"=w161) -> ("error out"=w158:errorcluster)  [unwired: 5 in, 2 out]
        n83 = call "UpdateUI.vi"("LabramHR References"=w151, "Acquisition Settings"=w150) -> ()  [unwired: 1 in]
        n84 = Unbundle By Name(w218) -> ("Status"=w219:refnum<notifier>)
        n85 = Not A Number/Path/Refnum?(number/path/refnum=w219) -> (NaN/Path/Refnum?=w220:bool)
        n86 = case shown="False" w220 {
          tunnel: [w226 w227] -> w190
          tunnel: w219 -> [w225 _]
          tunnel: w158 -> [w223 w227]
          frame False {
            n87 = Send Notification(notification="Status Updated", notifier=w225, error in (no error)=w223) -> (error out=w226:errorcluster)  [unwired: 1 out]
          }
          frame True {
          }
        }
      }
      frame "Load Configuration" {
        w236 = u16 0 items=["Don't show the setup dialog", "Show the setup, load the configuration", "Show the setup, don't load the configuration"] ("ShowDialog")
        n88 = call "Labspec LoadConfig.vi"("error in"=w238, "Path"=w231, "ShowDialog"=w236, "Automation Refnum In"=w230) -> ("error out"=w237:errorcluster)  [unwired: 7 out]
      }
      frame "Save Configuration" {
        w247 = u16 1 items=["Don't show the setup dialog", "Show the setup dialog"] ("ShowDialog")
        n89 = call "Labspec SaveConfig.vi"("error in"=w249, "Path"=w242, "ShowDialog"=w247, "Automation Refnum In"=w241) -> ("error out"=w248:errorcluster)  [unwired: 7 out]
      }
      frame "Acquire Spectrum" {
        w257 = T21 4 items=["Spectrum", "Image", "Spectrum (Labspec Parameters)", "Spectral Image", "Get Detector Temperature", "Real Time Acquisition", "Set Photomultiplier Parameter", "Macro Spot", "Cancel Acquisition", "Set Detector"] ("Mode")
        w281 = T21 0 items=["Spectrum", "Image", "Spectrum (Labspec Parameters)", "Spectral Image", "Get Detector Temperature", "Real Time Acquisition", "Set Photomultiplier Parameter", "Macro Spot", "Cancel Acquisition", "Set Detector"]  # Mode
        n90 = case shown="No Error" w295 {
          selector: w295 -> [w331 w335]
          tunnel: [w330 w334] -> w256
          tunnel: w278 -> [w326 w336]
          frame No Error {
            n91 = Unbundle By Name(w326) -> ("Instrument Status"=w327:refnum<vi>)
            n92 = control-ref of="Instrument Status"() -> (w329:refnum<vi>)
            n93 = Build Array(w327, w329) -> (w328:refnum<vi>[])
            n94 = call "Edit Status Indicator.vi"("error in (no error)"=w331, "State"=Instrument_Status_State."Measuring", "Instrument Status Refnum"=w328) -> ("error out"=w330:errorcluster)  [unwired: 1 in, 7 out]
          }
          frame Error {
            n95 = Unbundle By Name(w336) -> ("Instrument Status"=w337:refnum<vi>)
            n96 = control-ref of="Instrument Status"() -> (w339:refnum<vi>)
            n97 = Build Array(w337, w339) -> (w338:refnum<vi>[])
            n98 = call "Edit Status Indicator.vi"("State"=Instrument_Status_State."Unknown", "Instrument Status Refnum"=w338) -> ("error out"=w333:errorcluster)  [unwired: 2 in, 7 out]
            n99 = Merge Errors(w333, w335) -> (w334:errorcluster)
          }
        }
        n100 = Unbundle By Name(w293) -> ("Acquisition Mode"=w292:enum16{"Single Window", "Multi-Window"}, "Spectal Position (nm)"=w291:dbl, "From (nm)"=w288:dbl, "To (nm)"=w287:dbl, "Integration Time (s)"=w285:dbl, "Number of Accumulations"=w286:i32, "AutoScanning"=w284:bool, "Spike Removal"=w283:bool)
        n101 = case shown="\"Single Window\", Default" w292 {
          tunnel: w291 -> [w341 _]
          tunnel: [w341 w343] -> w290
          tunnel: [w341 w342] -> w289
          tunnel: w288 -> [_ w343]
          tunnel: w287 -> [_ w342]
          frame "Single Window", Default {
          }
          frame "Multi-Window" {
          }
        }
        n102 = case shown="True" w284 {
          tunnel: [w309 w310] -> w282
          frame True {
            w309 = T22 1000 items=[" "=0, "Auto Scanning"=1000, "Don't Close Shutter"=2000, "Accumulation Mode"=10000] ("Shutter Mode")
          }
          frame False {
            w310 = T22 0 items=[" "=0, "Auto Scanning"=1000, "Don't Close Shutter"=2000, "Accumulation Mode"=10000] ("Shutter Mode")
          }
        }
        n103 = case shown="True" w283 {
          tunnel: [w307 w308] -> w280
          frame True {
            w307 = T23 400 items=[" "=0, "Auto Show"=10, "No Spike Removing"=100, "Single Spike Removing"=200, "Double Spike Removing"=300, "Double Spike Removing with Autoadd"=400] ("Data Treatment")
          }
          frame False {
            w308 = T23 0 items=[" "=0, "Auto Show"=10, "No Spike Removing"=100, "Single Spike Removing"=200, "Double Spike Removing"=300, "Double Spike Removing with Autoadd"=400] ("Data Treatment")
          }
        }
        n104 = call "Labspec Acquire.vi"("Automation Refnum In"=w251, "Mode"=w257, "error in"=w256) -> ("Acq"=w252:i32, "error out"=w255:errorcluster)  [unwired: 9 in, 2 out]
        n105 = call "Labspec Acquire.vi"("Automation Refnum In"=w251, "From (nm)"=w290, "To (nm)"=w289, "Mode"=w281, "Shutter Mode"=w282, "Data Treatment"=w280, "error in"=w255, "Number of Accumulations"=w286, "Integration Time (s)"=w285) -> ("AcqID"=w259:i32, "error out"=w260:errorcluster)  [unwired: 3 in, 2 out]
        n106 = call "CalculateAxis.vi"("error in (no error)"=w260, "AcqID"=w259, "Automation Refnum in"=w251) -> ("error out"=w264:errorcluster, "Spectrum"=w258:T10)  [unwired: 7 in]
        n107 = Bundle By Name(cluster=w258, "Detector Temperature"=w252) -> (w253:T10)
        n108 = call "Clear Data.vi"("error in (no error)"=w264, "AcqID"=w259, "Automation Refnum in"=w251) -> ("error out"=w261:errorcluster)  [unwired: 8 in]
        n109 = Unbundle By Name(w278) -> ("Optical Spectrum Plot"=w279:T9)
        n110 = call "Plot Spectrum.vi"("Optical Spectrum Plot"=w279, "Optical Spectrum"=w265, "Spectrum"=w253, "error in (no error)"=w264) -> ("Optical Spectrum vs Energy"=w268:cluster{"data":dbl[], "data":dbl[]}, "Optical Spectrum vs Wavelength"=w267:cluster{"data":dbl[], "data":dbl[]}, "Optical Spectrum vs Raman Shift"=w266:cluster{"data":dbl[], "data":dbl[]}, "error out"=w263:errorcluster)  [unwired: 8 in]
        n111 = Merge Errors(w263, w261) -> (w262:errorcluster)
        n112 = Unbundle By Name(w272) -> ("Measurement"=w273:refnum<notifier>)
        n113 = Bundle By Name(cluster=w254, "Optical Spectrum vs Energy"=w268, "Optical Spectrum vs Wavelength"=w267, "Optical Spectrum vs Raman Shift"=w266) -> (w269:T20)
        n114 = Unbundle By Name(w272) -> ("Status"=w277:refnum<notifier>)
        n115 = case shown="No Error" w262 {
          selector: w262 -> [w316 w320]
          tunnel: [w315 w319] -> w294
          tunnel: w278 -> [w311 w321]
          frame No Error {
            n116 = Unbundle By Name(w311) -> ("Instrument Status"=w312:refnum<vi>)
            n117 = control-ref of="Instrument Status"() -> (w314:refnum<vi>)
            n118 = Build Array(w312, w314) -> (w313:refnum<vi>[])
            n119 = call "Edit Status Indicator.vi"("error in (no error)"=w316, "State"=Instrument_Status_State."Idle", "Instrument Status Refnum"=w313) -> ("error out"=w315:errorcluster)  [unwired: 1 in, 7 out]
          }
          frame Error {
            n120 = Unbundle By Name(w321) -> ("Instrument Status"=w322:refnum<vi>)
            n121 = control-ref of="Instrument Status"() -> (w324:refnum<vi>)
            n122 = Build Array(w322, w324) -> (w323:refnum<vi>[])
            n123 = call "Edit Status Indicator.vi"("State"=Instrument_Status_State."Unknown", "Instrument Status Refnum"=w323) -> ("error out"=w318:errorcluster)  [unwired: 2 in, 7 out]
            n124 = Merge Errors(w318, w320) -> (w319:errorcluster)
          }
        }
        n125 = Not A Number/Path/Refnum?(number/path/refnum=w273) -> (NaN/Path/Refnum?=w274:bool)
        n126 = case shown="False" w274 {
          tunnel: [w305 w306] -> w275
          tunnel: w273 -> [w304 _]
          tunnel: w253 -> [w303 _]
          tunnel: w262 -> [w302 w306]
          frame False {
            n127 = Send Notification(notification=w303, notifier=w304, error in (no error)=w302) -> (error out=w305:errorcluster)  [unwired: 1 out]
          }
          frame True {
          }
        }
        n128 = Not A Number/Path/Refnum?(number/path/refnum=w277) -> (NaN/Path/Refnum?=w276:bool)
        n129 = case shown="False" w276 {
          tunnel: w275 -> [w300 w301]
          tunnel: [w299 w301] -> w270
          tunnel: w277 -> [w298 _]
          frame False {
            n130 = Send Notification(notification="Measurement Performed", notifier=w298, error in (no error)=w300) -> (error out=w299:errorcluster)  [unwired: 1 out]
          }
          frame True {
          }
        }
        n131 = Merge Errors(w270, w294) -> (w271:errorcluster)
      }
      frame "Read File" {
        n132 = call "Labspec Load.vi"("error in"=w360, "Path"=w359, "Automation Refnum In"=w347) -> ("error out"=w349:errorcluster, "Data ID"=w348:i32)  [unwired: 7 out]
        n133 = call "Get Axis.vi"("error in (no error)"=w349, "AcqID"=w348, "Automation Refnum in"=w347) -> ("error out"=w345:errorcluster, "Spectrum"=w346:T10)  [unwired: 7 in]
        n134 = call "Clear Data.vi"("error in (no error)"=w345, "AcqID"=w348, "Automation Refnum in"=w347) -> ("error out"=w350:errorcluster)  [unwired: 8 in]
        n135 = Unbundle By Name(w369) -> ("Optical Spectrum Plot"=w370:T9)
        n136 = call "Plot Spectrum.vi"("Optical Spectrum Plot"=w370, "Optical Spectrum"=w353, "Spectrum"=w346, "error in (no error)"=w345) -> ("Optical Spectrum vs Energy"=w354:cluster{"data":dbl[], "data":dbl[]}, "Optical Spectrum vs Wavelength"=w355:cluster{"data":dbl[], "data":dbl[]}, "Optical Spectrum vs Raman Shift"=w356:cluster{"data":dbl[], "data":dbl[]}, "error out"=w352:errorcluster)  [unwired: 8 in]
        n137 = Merge Errors(w352, w350) -> (w351:errorcluster)
        n138 = Bundle By Name(cluster=w357, "Optical Spectrum vs Energy"=w354, "Optical Spectrum vs Wavelength"=w355, "Optical Spectrum vs Raman Shift"=w356) -> (w358:T20)
        n139 = Unbundle By Name(w363) -> ("Measurement"=w364:refnum<notifier>)
        n140 = Unbundle By Name(w363) -> ("Status"=w368:refnum<notifier>)
        n141 = case shown="No Error" w351 {
          selector: w351 -> [w388 w392]
          tunnel: [w387 w391] -> w371
          tunnel: w369 -> [w383 w393]
          frame No Error {
            n142 = Unbundle By Name(w383) -> ("Instrument Status"=w384:refnum<vi>)
            n143 = control-ref of="Instrument Status"() -> (w386:refnum<vi>)
            n144 = Build Array(w384, w386) -> (w385:refnum<vi>[])
            n145 = call "Edit Status Indicator.vi"("error in (no error)"=w388, "State"=Instrument_Status_State."Idle", "Instrument Status Refnum"=w385) -> ("error out"=w387:errorcluster)  [unwired: 1 in, 7 out]
          }
          frame Error {
            n146 = Unbundle By Name(w393) -> ("Instrument Status"=w394:refnum<vi>)
            n147 = control-ref of="Instrument Status"() -> (w396:refnum<vi>)
            n148 = Build Array(w394, w396) -> (w395:refnum<vi>[])
            n149 = call "Edit Status Indicator.vi"("State"=Instrument_Status_State."Unknown", "Instrument Status Refnum"=w395) -> ("error out"=w390:errorcluster)  [unwired: 2 in, 7 out]
            n150 = Merge Errors(w390, w392) -> (w391:errorcluster)
          }
        }
        n151 = Not A Number/Path/Refnum?(number/path/refnum=w364) -> (NaN/Path/Refnum?=w365:bool)
        n152 = case shown="False" w365 {
          tunnel: [w381 w382] -> w366
          tunnel: w364 -> [w380 _]
          tunnel: w346 -> [w379 _]
          tunnel: w351 -> [w378 w382]
          frame False {
            n153 = Send Notification(notification=w379, notifier=w380, error in (no error)=w378) -> (error out=w381:errorcluster)  [unwired: 1 out]
          }
          frame True {
          }
        }
        n154 = Not A Number/Path/Refnum?(number/path/refnum=w368) -> (NaN/Path/Refnum?=w367:bool)
        n155 = case shown="False" w367 {
          tunnel: w366 -> [w376 w377]
          tunnel: [w375 w377] -> w361
          tunnel: w368 -> [w374 _]
          frame False {
            n156 = Send Notification(notification="Measurement File Read", notifier=w374, error in (no error)=w376) -> (error out=w375:errorcluster)  [unwired: 1 out]
          }
          frame True {
          }
        }
        n157 = Merge Errors(w361, w371) -> (w362:errorcluster)
      }
      frame "Set Laser" {
        n158 = case shown="No Error" w414 {
          selector: w414 -> [w444 w448]
          tunnel: [w443 w447] -> w413
          tunnel: w399 -> [w439 w449]
          frame No Error {
            n159 = Unbundle By Name(w439) -> ("Instrument Status"=w440:refnum<vi>)
            n160 = control-ref of="Instrument Status"() -> (w442:refnum<vi>)
            n161 = Build Array(w440, w442) -> (w441:refnum<vi>[])
            n162 = call "Edit Status Indicator.vi"("error in (no error)"=w444, "State"=Instrument_Status_State."Configuring", "Instrument Status Refnum"=w441) -> ("error out"=w443:errorcluster)  [unwired: 1 in, 7 out]
          }
          frame Error {
            n163 = Unbundle By Name(w449) -> ("Instrument Status"=w450:refnum<vi>)
            n164 = control-ref of="Instrument Status"() -> (w452:refnum<vi>)
            n165 = Build Array(w450, w452) -> (w451:refnum<vi>[])
            n166 = call "Edit Status Indicator.vi"("State"=Instrument_Status_State."Unknown", "Instrument Status Refnum"=w451) -> ("error out"=w446:errorcluster)  [unwired: 2 in, 7 out]
            n167 = Merge Errors(w446, w448) -> (w447:errorcluster)
          }
        }
        n168 = Unbundle By Name(w402) -> ("Laser Wavelength"=w401:T6)
        n169 = Unbundle By Name(w399) -> ("Laser"=w400:refnum<vi>)
        n170 = call "LabramHR MotorControl.vi"("Control Refnum"=w400, "error in"=w413, "Destination"=w401, "Motor Name"=MoveMotor_Motor_Name."Laser", "Automation Refnum In"=w410) -> ("error out"=w405:errorcluster, "MotorID"=w417:i32)  [unwired: 1 in, 4 out]
        n171 = Bundle By Name(cluster=w416, "Laser"=w417) -> (w415:T11)
        n172 = case shown="No Error" w405 {
          selector: w405 -> [w429 w433]
          tunnel: [w428 w432] -> w412
          tunnel: w399 -> [w424 w434]
          frame No Error {
            n173 = Unbundle By Name(w424) -> ("Instrument Status"=w425:refnum<vi>)
            n174 = control-ref of="Instrument Status"() -> (w427:refnum<vi>)
            n175 = Build Array(w425, w427) -> (w426:refnum<vi>[])
            n176 = call "Edit Status Indicator.vi"("error in (no error)"=w429, "State"=Instrument_Status_State."Idle", "Instrument Status Refnum"=w426) -> ("error out"=w428:errorcluster)  [unwired: 1 in, 7 out]
          }
          frame Error {
            n177 = Unbundle By Name(w434) -> ("Instrument Status"=w435:refnum<vi>)
            n178 = control-ref of="Instrument Status"() -> (w437:refnum<vi>)
            n179 = Build Array(w435, w437) -> (w436:refnum<vi>[])
            n180 = call "Edit Status Indicator.vi"("State"=Instrument_Status_State."Unknown", "Instrument Status Refnum"=w436) -> ("error out"=w431:errorcluster)  [unwired: 2 in, 7 out]
            n181 = Merge Errors(w431, w433) -> (w432:errorcluster)
          }
        }
        n182 = Unbundle By Name(w406) -> ("Status"=w407:refnum<notifier>)
        n183 = Not A Number/Path/Refnum?(number/path/refnum=w407) -> (NaN/Path/Refnum?=w408:bool)
        n184 = case shown="False" w408 {
          tunnel: w405 -> [w422 w423]
          tunnel: [w421 w423] -> w403
          tunnel: w407 -> [w420 _]
          frame False {
            n185 = Send Notification(notification="Laser Configured", notifier=w420, error in (no error)=w422) -> (error out=w421:errorcluster)  [unwired: 1 out]
          }
          frame True {
          }
        }
        n186 = Merge Errors(w403, w412) -> (w404:errorcluster)
      }
      frame "Set Filter" {
        # "Check values for Filter"
        n187 = case shown="No Error" w470 {
          selector: w470 -> [w500 w504]
          tunnel: [w499 w503] -> w469
          tunnel: w456 -> [w495 w505]
          frame No Error {
            n188 = Unbundle By Name(w495) -> ("Instrument Status"=w496:refnum<vi>)
            n189 = control-ref of="Instrument Status"() -> (w498:refnum<vi>)
            n190 = Build Array(w496, w498) -> (w497:refnum<vi>[])
            n191 = call "Edit Status Indicator.vi"("error in (no error)"=w500, "State"=Instrument_Status_State."Configuring", "Instrument Status Refnum"=w497) -> ("error out"=w499:errorcluster)  [unwired: 1 in, 7 out]
          }
          frame Error {
            n192 = Unbundle By Name(w505) -> ("Instrument Status"=w506:refnum<vi>)
            n193 = control-ref of="Instrument Status"() -> (w508:refnum<vi>)
            n194 = Build Array(w506, w508) -> (w507:refnum<vi>[])
            n195 = call "Edit Status Indicator.vi"("State"=Instrument_Status_State."Unknown", "Instrument Status Refnum"=w507) -> ("error out"=w502:errorcluster)  [unwired: 2 in, 7 out]
            n196 = Merge Errors(w502, w504) -> (w503:errorcluster)
          }
        }
        n197 = Unbundle By Name(w458) -> ("Neutral Density Filter"=w457:T7)
        n198 = Unbundle By Name(w456) -> ("Filter"=w455:refnum<vi>)
        n199 = call "LabramHR MotorControl.vi"("Control Refnum"=w455, "error in"=w469, "Destination"=w457, "Motor Name"=MoveMotor_Motor_Name."Filter", "Automation Refnum In"=w466) -> ("error out"=w460:errorcluster, "MotorID"=w474:i32)  [unwired: 1 in, 4 out]
        n200 = Bundle By Name(cluster=w473, "Filter"=w474) -> (w472:T11)
        n201 = case shown="No Error" w460 {
          selector: w460 -> [w485 w489]
          tunnel: [w484 w488] -> w468
          tunnel: w456 -> [w480 w490]
          frame No Error {
            n202 = Unbundle By Name(w480) -> ("Instrument Status"=w481:refnum<vi>)
            n203 = control-ref of="Instrument Status"() -> (w483:refnum<vi>)
            n204 = Build Array(w481, w483) -> (w482:refnum<vi>[])
            n205 = call "Edit Status Indicator.vi"("error in (no error)"=w485, "State"=Instrument_Status_State."Idle", "Instrument Status Refnum"=w482) -> ("error out"=w484:errorcluster)  [unwired: 1 in, 7 out]
          }
          frame Error {
            n206 = Unbundle By Name(w490) -> ("Instrument Status"=w491:refnum<vi>)
            n207 = control-ref of="Instrument Status"() -> (w493:refnum<vi>)
            n208 = Build Array(w491, w493) -> (w492:refnum<vi>[])
            n209 = call "Edit Status Indicator.vi"("State"=Instrument_Status_State."Unknown", "Instrument Status Refnum"=w492) -> ("error out"=w487:errorcluster)  [unwired: 2 in, 7 out]
            n210 = Merge Errors(w487, w489) -> (w488:errorcluster)
          }
        }
        n211 = Unbundle By Name(w459) -> ("Status"=w463:refnum<notifier>)
        n212 = Not A Number/Path/Refnum?(number/path/refnum=w463) -> (NaN/Path/Refnum?=w464:bool)
        n213 = case shown="True" w464 {
          tunnel: w460 -> [w478 w479]
          tunnel: [w477 w479] -> w461
          tunnel: w463 -> [w476 _]
          frame False {
            n214 = Send Notification(notification="Filter Configured", notifier=w476, error in (no error)=w478) -> (error out=w477:errorcluster)  [unwired: 1 out]
          }
          frame True {
          }
        }
        n215 = Merge Errors(w461, w468) -> (w462:errorcluster)
      }
      frame "Set Hole" {
        n216 = case shown="No Error" w525 {
          selector: w525 -> [w556 w560]
          tunnel: [w555 w559] -> w524
          tunnel: w526 -> [w551 w561]
          frame No Error {
            n217 = Unbundle By Name(w551) -> ("Instrument Status"=w552:refnum<vi>)
            n218 = control-ref of="Instrument Status"() -> (w554:refnum<vi>)
            n219 = Build Array(w552, w554) -> (w553:refnum<vi>[])
            n220 = call "Edit Status Indicator.vi"("error in (no error)"=w556, "State"=Instrument_Status_State."Configuring", "Instrument Status Refnum"=w553) -> ("error out"=w555:errorcluster)  [unwired: 1 in, 7 out]
          }
          frame Error {
            n221 = Unbundle By Name(w561) -> ("Instrument Status"=w562:refnum<vi>)
            n222 = control-ref of="Instrument Status"() -> (w564:refnum<vi>)
            n223 = Build Array(w562, w564) -> (w563:refnum<vi>[])
            n224 = call "Edit Status Indicator.vi"("State"=Instrument_Status_State."Unknown", "Instrument Status Refnum"=w563) -> ("error out"=w558:errorcluster)  [unwired: 2 in, 7 out]
            n225 = Merge Errors(w558, w560) -> (w559:errorcluster)
          }
        }
        n226 = Unbundle By Name(w512) -> ("Confocal Hole Size (µm)"=w511:dbl)
        n227 = Unbundle By Name(w526) -> ("Hole"=w513:refnum<vi>)
        n228 = call "LabramHR MotorControl.vi"("Control Refnum"=w513, "error in"=w524, "Destination"=w511, "Motor Name"=MoveMotor_Motor_Name."Hole", "Automation Refnum In"=w521) -> ("error out"=w516:errorcluster, "MotorID"=w530:i32)  [unwired: 1 in, 4 out]
        n229 = Bundle By Name(cluster=w529, "Hole"=w530) -> (w528:T11)
        n230 = case shown="No Error" w516 {
          selector: w516 -> [w541 w545]
          tunnel: [w540 w544] -> w523
          tunnel: w526 -> [w536 w546]
          frame No Error {
            n231 = Unbundle By Name(w536) -> ("Instrument Status"=w537:refnum<vi>)
            n232 = control-ref of="Instrument Status"() -> (w539:refnum<vi>)
            n233 = Build Array(w537, w539) -> (w538:refnum<vi>[])
            n234 = call "Edit Status Indicator.vi"("error in (no error)"=w541, "State"=Instrument_Status_State."Idle", "Instrument Status Refnum"=w538) -> ("error out"=w540:errorcluster)  [unwired: 1 in, 7 out]
          }
          frame Error {
            n235 = Unbundle By Name(w546) -> ("Instrument Status"=w547:refnum<vi>)
            n236 = control-ref of="Instrument Status"() -> (w549:refnum<vi>)
            n237 = Build Array(w547, w549) -> (w548:refnum<vi>[])
            n238 = call "Edit Status Indicator.vi"("State"=Instrument_Status_State."Unknown", "Instrument Status Refnum"=w548) -> ("error out"=w543:errorcluster)  [unwired: 2 in, 7 out]
            n239 = Merge Errors(w543, w545) -> (w544:errorcluster)
          }
        }
        n240 = Unbundle By Name(w514) -> ("Status"=w518:refnum<notifier>)
        n241 = Not A Number/Path/Refnum?(number/path/refnum=w518) -> (NaN/Path/Refnum?=w519:bool)
        n242 = case shown="False" w519 {
          tunnel: w516 -> [w534 w535]
          tunnel: [w533 w535] -> w515
          tunnel: w518 -> [w532 _]
          frame False {
            n243 = Send Notification(notification="Confocal Hole Configured", notifier=w532, error in (no error)=w534) -> (error out=w533:errorcluster)  [unwired: 1 out]
          }
          frame True {
          }
        }
        n244 = Merge Errors(w515, w523) -> (w517:errorcluster)
      }
      frame "Set Grating" {
        n245 = case shown="No Error" w591 {
          selector: w591 -> [w606 w610]
          tunnel: [w605 w609] -> w590
          tunnel: w577 -> [w601 w611]
          frame No Error {
            n246 = Unbundle By Name(w601) -> ("Instrument Status"=w602:refnum<vi>)
            n247 = control-ref of="Instrument Status"() -> (w604:refnum<vi>)
            n248 = Build Array(w602, w604) -> (w603:refnum<vi>[])
            n249 = call "Edit Status Indicator.vi"("error in (no error)"=w606, "State"=Instrument_Status_State."Configuring", "Instrument Status Refnum"=w603) -> ("error out"=w605:errorcluster)  [unwired: 1 in, 7 out]
          }
          frame Error {
            n250 = Unbundle By Name(w611) -> ("Instrument Status"=w612:refnum<vi>)
            n251 = control-ref of="Instrument Status"() -> (w614:refnum<vi>)
            n252 = Build Array(w612, w614) -> (w613:refnum<vi>[])
            n253 = call "Edit Status Indicator.vi"("State"=Instrument_Status_State."Unknown", "Instrument Status Refnum"=w613) -> ("error out"=w608:errorcluster)  [unwired: 2 in, 7 out]
            n254 = Merge Errors(w608, w610) -> (w609:errorcluster)
          }
        }
        n255 = Unbundle By Name(w577) -> ("Spectal Position"=w567:refnum<vi>, "Grating"=w579:refnum<vi>)
        n256 = Unbundle By Name(w581) -> ("Grating"=w580:T3)
        n257 = call "LabramHR MotorControl.vi"("Control Refnum"=w579, "error in"=w590, "Destination"=w580, "Motor Name"=MoveMotor_Motor_Name."Grating", "Automation Refnum In"=w576) -> ("error out"=w575:errorcluster, "MotorID"=w595:i32)  [unwired: 1 in, 4 out]
        n258 = Bundle By Name(cluster=w594, "Grating"=w595) -> (w593:T11)
        n259 = Unbundle By Name(w571) -> ("Spectal Position (nm)"=w570:dbl)
        n260 = call "Spectrometer GetControlPosition.vi"("error in"=w575, "Control Refnum"=w567, "Motor Name"=MoveMotor_Motor_Name."Spectro", "Automation Refnum In"=w576) -> ("error out"=w573:errorcluster, "Position"=w568:variant)  [unwired: 5 in, 1 out]
        n261 = Variant To Data(error in=w573, type=w570, Variant=w568) -> (data=w569:dbl, error out=w574:errorcluster)
        n262 = property on="Spectal Position (nm)" class="DigNum (strict)"(error in=w574, "Value"=w569) -> (error out=w572:errorcluster)  [unwired: 1 in, 1 out]
        n263 = Unbundle By Name(w582) -> ("Status"=w584:refnum<notifier>)
        n264 = case shown="No Error" w572 {
          selector: w572 -> [w621 w625]
          tunnel: [w620 w624] -> w589
          tunnel: w577 -> [w616 w626]
          frame No Error {
            n265 = Unbundle By Name(w616) -> ("Instrument Status"=w617:refnum<vi>)
            n266 = control-ref of="Instrument Status"() -> (w619:refnum<vi>)
            n267 = Build Array(w617, w619) -> (w618:refnum<vi>[])
            n268 = call "Edit Status Indicator.vi"("error in (no error)"=w621, "State"=Instrument_Status_State."Idle", "Instrument Status Refnum"=w618) -> ("error out"=w620:errorcluster)  [unwired: 1 in, 7 out]
          }
          frame Error {
            n269 = Unbundle By Name(w626) -> ("Instrument Status"=w627:refnum<vi>)
            n270 = control-ref of="Instrument Status"() -> (w629:refnum<vi>)
            n271 = Build Array(w627, w629) -> (w628:refnum<vi>[])
            n272 = call "Edit Status Indicator.vi"("State"=Instrument_Status_State."Unknown", "Instrument Status Refnum"=w628) -> ("error out"=w623:errorcluster)  [unwired: 2 in, 7 out]
            n273 = Merge Errors(w623, w625) -> (w624:errorcluster)
          }
        }
        n274 = Not A Number/Path/Refnum?(number/path/refnum=w584) -> (NaN/Path/Refnum?=w585:bool)
        n275 = case shown="False" w585 {
          tunnel: w572 -> [w599 w600]
          tunnel: [w598 w600] -> w583
          tunnel: w584 -> [w597 _]
          frame False {
            n276 = Send Notification(notification="Grating Configured", notifier=w597, error in (no error)=w599) -> (error out=w598:errorcluster)  [unwired: 1 out]
          }
          frame True {
          }
        }
        n277 = Merge Errors(w583, w589) -> (w586:errorcluster)
      }
      frame "Set Grating Position" {
        n278 = case shown="No Error" w647 {
          selector: w647 -> [w677 w681]
          tunnel: [w676 w680] -> w646
          tunnel: w644 -> [w672 w682]
          frame No Error {
            n279 = Unbundle By Name(w672) -> ("Instrument Status"=w673:refnum<vi>)
            n280 = control-ref of="Instrument Status"() -> (w675:refnum<vi>)
            n281 = Build Array(w673, w675) -> (w674:refnum<vi>[])
            n282 = call "Edit Status Indicator.vi"("error in (no error)"=w677, "State"=Instrument_Status_State."Configuring", "Instrument Status Refnum"=w674) -> ("error out"=w676:errorcluster)  [unwired: 1 in, 7 out]
          }
          frame Error {
            n283 = Unbundle By Name(w682) -> ("Instrument Status"=w683:refnum<vi>)
            n284 = control-ref of="Instrument Status"() -> (w685:refnum<vi>)
            n285 = Build Array(w683, w685) -> (w684:refnum<vi>[])
            n286 = call "Edit Status Indicator.vi"("State"=Instrument_Status_State."Unknown", "Instrument Status Refnum"=w684) -> ("error out"=w679:errorcluster)  [unwired: 2 in, 7 out]
            n287 = Merge Errors(w679, w681) -> (w680:errorcluster)
          }
        }
        n288 = Unbundle By Name(w633) -> ("Spectal Position (nm)"=w632:dbl)
        n289 = Unbundle By Name(w644) -> ("Spectal Position"=w634:refnum<vi>)
        n290 = call "LabramHR MotorControl.vi"("Control Refnum"=w634, "error in"=w646, "Destination"=w632, "Motor Name"=MoveMotor_Motor_Name."Spectro", "Automation Refnum In"=w642) -> ("error out"=w636:errorcluster, "MotorID"=w651:i32)  [unwired: 1 in, 4 out]
        n291 = Bundle By Name(cluster=w650, "Spectro"=w651) -> (w649:T11)
        n292 = case shown="No Error" w636 {
          selector: w636 -> [w662 w667]
          tunnel: [w661 w666] -> w645
          tunnel: w644 -> [w657 w664]
          frame No Error {
            n293 = Unbundle By Name(w657) -> ("Instrument Status"=w658:refnum<vi>)
            n294 = control-ref of="Instrument Status"() -> (w660:refnum<vi>)
            n295 = Build Array(w658, w660) -> (w659:refnum<vi>[])
            n296 = call "Edit Status Indicator.vi"("error in (no error)"=w662, "State"=Instrument_Status_State."Idle", "Instrument Status Refnum"=w659) -> ("error out"=w661:errorcluster)  [unwired: 1 in, 7 out]
          }
          frame Error {
            n297 = Unbundle By Name(w664) -> ("Instrument Status"=w668:refnum<vi>)
            n298 = control-ref of="Instrument Status"() -> (w670:refnum<vi>)
            n299 = Build Array(w668, w670) -> (w669:refnum<vi>[])
            n300 = call "Edit Status Indicator.vi"("State"=Instrument_Status_State."Unknown", "Instrument Status Refnum"=w669) -> ("error out"=w665:errorcluster)  [unwired: 2 in, 7 out]
            n301 = Merge Errors(w665, w667) -> (w666:errorcluster)
          }
        }
        n302 = Unbundle By Name(w635) -> ("Status"=w638:refnum<notifier>)
        n303 = Not A Number/Path/Refnum?(number/path/refnum=w638) -> (NaN/Path/Refnum?=w639:bool)
        n304 = case shown="False" w639 {
          tunnel: w636 -> [w655 w656]
          tunnel: [w654 w656] -> w637
          tunnel: w638 -> [w653 _]
          frame False {
            n305 = Send Notification(notification="Spectral Position Configured", notifier=w653, error in (no error)=w655) -> (error out=w654:errorcluster)  [unwired: 1 out]
          }
          frame True {
          }
        }
        n306 = Merge Errors(w637, w645) -> (w640:errorcluster)
      }
      frame "Set Detector" {
        w696 = T21 4 items=["Spectrum", "Image", "Spectrum (Labspec Parameters)", "Spectral Image", "Get Detector Temperature", "Real Time Acquisition", "Set Photomultiplier Parameter", "Macro Spot", "Cancel Acquisition", "Set Detector"] ("Mode")
        n307 = case shown="No Error" w710 {
          selector: w710 -> [w745 w749]
          tunnel: [w744 w748] -> w709
          tunnel: w692 -> [w740 w750]
          frame No Error {
            n308 = Unbundle By Name(w740) -> ("Instrument Status"=w741:refnum<vi>)
            n309 = control-ref of="Instrument Status"() -> (w743:refnum<vi>)
            n310 = Build Array(w741, w743) -> (w742:refnum<vi>[])
            n311 = call "Edit Status Indicator.vi"("error in (no error)"=w745, "State"=Instrument_Status_State."Configuring", "Instrument Status Refnum"=w742) -> ("error out"=w744:errorcluster)  [unwired: 1 in, 7 out]
          }
          frame Error {
            n312 = Unbundle By Name(w750) -> ("Instrument Status"=w751:refnum<vi>)
            n313 = control-ref of="Instrument Status"() -> (w753:refnum<vi>)
            n314 = Build Array(w751, w753) -> (w752:refnum<vi>[])
            n315 = call "Edit Status Indicator.vi"("State"=Instrument_Status_State."Unknown", "Instrument Status Refnum"=w752) -> ("error out"=w747:errorcluster)  [unwired: 2 in, 7 out]
            n316 = Merge Errors(w747, w749) -> (w748:errorcluster)
          }
        }
        n317 = Unbundle By Name(w692) -> ("Detector"=w698:refnum<vi>)
        n318 = Unbundle By Name(w692) -> ("Optical Spectrum Plot.Detector Temperature"=w688:refnum<vi>)
        n319 = Unbundle By Name(w706) -> ("Detector"=w705:T4)
        n320 = call "LabramHR MotorControl.vi"("Control Refnum"=w698, "error in"=w709, "Destination"=w705, "Motor Name"=MoveMotor_Motor_Name."Detector", "Automation Refnum In"=w695) -> ("error out"=w694:errorcluster, "MotorID"=w714:i32)  [unwired: 1 in, 4 out]
        n321 = call "Labspec Acquire.vi"("Automation Refnum In"=w695, "Mode"=w696, "error in"=w694) -> ("Acq"=w690:i32, "error out"=w693:errorcluster)  [unwired: 9 in, 2 out]
        n322 = Bundle By Name(cluster=w704, "Detector Temperature"=w690) -> (w697:T10)
        n323 = Not A Number/Path/Refnum?(number/path/refnum=w688) -> (NaN/Path/Refnum?=w689:bool)
        n324 = Bundle By Name(cluster=w713, "Spectro"=w714) -> (w712:T11)
        n325 = case shown="False" w689 {
          tunnel: w693 -> [w718 w719]
          tunnel: [w717 w719] -> w691
          tunnel: w688 -> [w716 _]
          tunnel: w690 -> [w715 _]
          frame False {
            n326 = property class="DigNum (strict)"(reference=w716, error in=w718, "Value"=w715) -> (error out=w717:errorcluster)  [unwired: 1 out]
          }
          frame True {
          }
        }
        n327 = Unbundle By Name(w700) -> ("Status"=w701:refnum<notifier>)
        n328 = case shown="No Error" w691 {
          selector: w691 -> [w730 w735]
          tunnel: [w729 w734] -> w708
          tunnel: w692 -> [w725 w732]
          frame No Error {
            n329 = Unbundle By Name(w725) -> ("Instrument Status"=w726:refnum<vi>)
            n330 = control-ref of="Instrument Status"() -> (w728:refnum<vi>)
            n331 = Build Array(w726, w728) -> (w727:refnum<vi>[])
            n332 = call "Edit Status Indicator.vi"("error in (no error)"=w730, "State"=Instrument_Status_State."Idle", "Instrument Status Refnum"=w727) -> ("error out"=w729:errorcluster)  [unwired: 1 in, 7 out]
          }
          frame Error {
            n333 = Unbundle By Name(w732) -> ("Instrument Status"=w736:refnum<vi>)
            n334 = control-ref of="Instrument Status"() -> (w738:refnum<vi>)
            n335 = Build Array(w736, w738) -> (w737:refnum<vi>[])
            n336 = call "Edit Status Indicator.vi"("State"=Instrument_Status_State."Unknown", "Instrument Status Refnum"=w737) -> ("error out"=w733:errorcluster)  [unwired: 2 in, 7 out]
            n337 = Merge Errors(w733, w735) -> (w734:errorcluster)
          }
        }
        n338 = Not A Number/Path/Refnum?(number/path/refnum=w701) -> (NaN/Path/Refnum?=w702:bool)
        n339 = case shown="False" w702 {
          tunnel: w691 -> [w723 w724]
          tunnel: [w722 w724] -> w699
          tunnel: w701 -> [w721 _]
          frame False {
            n340 = Send Notification(notification="Detector Configured", notifier=w721, error in (no error)=w723) -> (error out=w722:errorcluster)  [unwired: 1 out]
          }
          frame True {
          }
        }
        n341 = Merge Errors(w699, w708) -> (w703:errorcluster)
      }
      frame "Set Acquisition Mode" {
        n342 = Unbundle By Name(w764) -> ("Acquisition Mode"=w763:enum16{"Single Window", "Multi-Window"})
        n343 = case shown="\"Single Window\", Default" w763 {
          tunnel: [T19."Enabled" ("Disabled") T19."Disabled and Grayed Out" ("Disabled")] -> w766
          tunnel: [T19."Disabled and Grayed Out" ("Disabled") T19."Enabled" ("Disabled")] -> w765
          tunnel: [enum32{"Single", "Multi-Window"}."Multi-Window" ("Value") enum32{"Single", "Multi-Window"}."Single" ("Value")] -> w755
          frame "Multi-Window" {
          }
          frame "Single Window", Default {
          }
        }
        n344 = Unbundle By Name(w757) -> ("Spectal Position"=w769:refnum<vi>, "From"=w768:refnum<vi>, "To"=w767:refnum<vi>)
        n345 = control-ref of="Spectal Position (nm)"() -> (w773:refnum<vi>)
        n346 = control-ref of="To (nm)"() -> (w770:refnum<vi>)
        n347 = control-ref of="From (nm)"() -> (w771:refnum<vi>)
        n348 = Build Array(w765, w766, w766, w765, w766, w766) -> (w762:T24)
        n349 = Build Array(w773, w771, w770, w769, w768, w767) -> (w772:refnum<vi>[])
        n350 = for {
          tunnel: w772 -> [w792] mode=indexing
          shift-right: [w793] -> w759
          shift-left: w774 -> [w794]
          tunnel: w762 -> [w791] mode=indexing
          n351 = Not A Number/Path/Refnum?(number/path/refnum=w792) -> (NaN/Path/Refnum?=w795:bool)
          n352 = case shown="False" w795 {
            tunnel: w794 -> [w799 w800]
            tunnel: [w798 w800] -> w793
            tunnel: w792 -> [w797 _]
            tunnel: w791 -> [w796 _]
            frame False {
              n353 = property class="DigNum (strict)"(reference=w797, error in=w799, "DisabledEnum"=w796) -> (error out=w798:errorcluster)  [unwired: 1 out]
            }
            frame True {
            }
          }
        }
        n354 = Unbundle By Name(w757) -> ("Acquisition Mode Panel"=w756:refnum<vi>)
        n355 = Not A Number/Path/Refnum?(number/path/refnum=w756) -> (NaN/Path/Refnum?=w760:bool)
        n356 = case shown="False" w760 {
          tunnel: w759 -> [w783 w784]
          tunnel: [w782 w784] -> w758
          tunnel: w756 -> [w781 _]
          tunnel: w755 -> [w780 _]
          frame False {
            n357 = property class="TabCtl (strict)"(reference=w781, error in=w783, "Value"=w780) -> (error out=w782:errorcluster)  [unwired: 1 out]
          }
          frame True {
          }
        }
      }
      frame "Update Refnums" {
        n358 = Unbundle By Name("Labram HR Notifications") -> ("Status"=w807:refnum<notifier>)
        n359 = Not A Number/Path/Refnum?(number/path/refnum=w807) -> (NaN/Path/Refnum?=w808:bool)
        n360 = case shown="False" w808 {
          tunnel: w805 -> [w815 w816]
          tunnel: [w814 w816] -> w804
          tunnel: w807 -> [w813 _]
          frame False {
            n361 = Send Notification(notification="Refnums Updated", notifier=w813, error in (no error)=w815) -> (error out=w814:errorcluster)  [unwired: 1 out]
          }
          frame True {
          }
        }
      }
      frame "Disconnect", Default {
        n362 = case shown="No Error" w827 {
          selector: w827 -> [w873 w877]
          tunnel: [w872 w876] -> w826
          tunnel: w823 -> [w868 w878]
          frame No Error {
            n363 = Unbundle By Name(w868) -> ("Instrument Status"=w869:refnum<vi>)
            n364 = control-ref of="Instrument Status"() -> (w871:refnum<vi>)
            n365 = Build Array(w869, w871) -> (w870:refnum<vi>[])
            n366 = call "Edit Status Indicator.vi"("error in (no error)"=w873, "State"=Instrument_Status_State."Disconnected", "Instrument Status Refnum"=w870) -> ("error out"=w872:errorcluster)  [unwired: 1 in, 7 out]
          }
          frame Error {
            n367 = Unbundle By Name(w878) -> ("Instrument Status"=w879:refnum<vi>)
            n368 = control-ref of="Instrument Status"() -> (w881:refnum<vi>)
            n369 = Build Array(w879, w881) -> (w880:refnum<vi>[])
            n370 = call "Edit Status Indicator.vi"("State"=Instrument_Status_State."Unknown", "Instrument Status Refnum"=w880) -> ("error out"=w875:errorcluster)  [unwired: 2 in, 7 out]
            n371 = Merge Errors(w875, w877) -> (w876:errorcluster)
          }
        }
        n372 = Unbundle By Name(w830) -> ("Spectrometer Settings.Grating"=w838:T3, "Spectrometer Settings.Confocal Hole Size (µm)"=w839:dbl, "Spectrometer Settings.Detector"=w831:T4)
        n373 = Unbundle By Name(w830) -> ("Acquisition Settings.Spectal Position (nm)"=w837:dbl)
        n374 = Unbundle By Name(w830) -> ("Laser Settings.Neutral Density Filter"=w840:T7, "Laser Settings.Laser Wavelength"=w841:T6)
        n375 = Unbundle By Name(w823) -> ("Spectal Position"=w817:refnum<vi>, "Detector"=w818:refnum<vi>, "Grating"=w819:refnum<vi>, "Hole"=w820:refnum<vi>, "Filter"=w821:refnum<vi>, "Laser"=w822:refnum<vi>)
        n376 = call "LabramHR MotorControl.vi"("Control Refnum"=w822, "error in"=w826, "Destination"=w841, "Motor Name"=MoveMotor_Motor_Name."Laser", "Automation Refnum In"=w824) -> ("error out"=w857:errorcluster, "MotorID"=w847:i32)  [unwired: 1 in, 4 out]
        n377 = Bundle By Name(cluster=w829, "Laser"=w847) -> (w856:T11)
        n378 = call "LabramHR MotorControl.vi"("Control Refnum"=w821, "error in"=w857, "Destination"=w840, "Motor Name"=MoveMotor_Motor_Name."Filter", "Automation Refnum In"=w824) -> ("error out"=w855:errorcluster, "MotorID"=w858:i32)  [unwired: 1 in, 4 out]
        n379 = Bundle By Name(cluster=w856, "Filter"=w858) -> (w850:T11)
        n380 = call "LabramHR MotorControl.vi"("Control Refnum"=w820, "error in"=w855, "Destination"=w839, "Motor Name"=MoveMotor_Motor_Name."Hole", "Automation Refnum In"=w824) -> ("error out"=w853:errorcluster, "MotorID"=w854:i32)  [unwired: 1 in, 4 out]
        n381 = Bundle By Name(cluster=w850, "Hole"=w854) -> (w849:T11)
        n382 = call "LabramHR MotorControl.vi"("Control Refnum"=w819, "error in"=w853, "Destination"=w838, "Motor Name"=MoveMotor_Motor_Name."Grating", "Automation Refnum In"=w824) -> ("error out"=w836:errorcluster, "MotorID"=w851:i32)  [unwired: 1 in, 4 out]
        n383 = Bundle By Name(cluster=w849, "Grating"=w851) -> (w848:T11)
        n384 = call "LabramHR MotorControl.vi"("Control Refnum"=w818, "error in"=w836, "Destination"=w831, "Motor Name"=MoveMotor_Motor_Name."Detector", "Automation Refnum In"=w824) -> ("error out"=w835:errorcluster, "MotorID"=w833:i32)  [unwired: 1 in, 4 out]
        n385 = Bundle By Name(cluster=w848, "Detector"=w833) -> (w834:T11)
        n386 = call "LabramHR MotorControl.vi"("Control Refnum"=w817, "error in"=w835, "Destination"=w837, "Motor Name"=MoveMotor_Motor_Name."Spectro", "Automation Refnum In"=w824) -> ("error out"=w825:errorcluster, "MotorID"=w852:i32)  [unwired: 1 in, 4 out]
        n387 = Bundle By Name(cluster=w834, "Spectro"=w852) -> (w828:T11)
        n388 = call "Labspec CloseCom.vi"("error in"=w825, "Automation Refnum In"=w824) -> ("error out"=w860:errorcluster)  [unwired: 9 out]
        n389 = case shown="No Error" w860 {
          selector: w860 -> [w893 w897]
          tunnel: [w892 w896] -> w861
          tunnel: w823 -> [w888 w898]
          frame No Error {
            n390 = Unbundle By Name(w888) -> ("Instrument Status"=w889:refnum<vi>)
            n391 = control-ref of="Instrument Status"() -> (w891:refnum<vi>)
            n392 = Build Array(w889, w891) -> (w890:refnum<vi>[])
            n393 = call "Edit Status Indicator.vi"("error in (no error)"=w893, "State"=Instrument_Status_State."Disconnected", "Instrument Status Refnum"=w890) -> ("error out"=w892:errorcluster)  [unwired: 1 in, 7 out]
          }
          frame Error {
            n394 = Unbundle By Name(w898) -> ("Instrument Status"=w899:refnum<vi>)
            n395 = control-ref of="Instrument Status"() -> (w901:refnum<vi>)
            n396 = Build Array(w899, w901) -> (w900:refnum<vi>[])
            n397 = call "Edit Status Indicator.vi"("State"=Instrument_Status_State."Unknown", "Instrument Status Refnum"=w900) -> ("error out"=w895:errorcluster)  [unwired: 2 in, 7 out]
            n398 = Merge Errors(w895, w897) -> (w896:errorcluster)
          }
        }
        n399 = Unbundle By Name(w864) -> ("Status"=w865:refnum<notifier>)
        n400 = Not A Number/Path/Refnum?(number/path/refnum=w865) -> (NaN/Path/Refnum?=w866:bool)
        n401 = case shown="False" w866 {
          tunnel: w860 -> [w886 w887]
          tunnel: [w885 w887] -> w863
          tunnel: w865 -> [w884 _]
          frame False {
            n402 = Send Notification(notification="Disconnected", notifier=w884, error in (no error)=w886) -> (error out=w885:errorcluster)  [unwired: 1 out]
          }
          frame True {
          }
        }
        n403 = Merge Errors(w863, w861) -> (w862:errorcluster)
      }
    }
  }
  "error out" <- w13
  "Motor ID" <- w7
  "Spectrum" <- w6
  n404 = Unbundle By Name(w5) -> ("Optical Spectrum vs Energy"=→"Optical Spectrum vs Energy":cluster{"Intensity":dbl[], "Energy":dbl[]}, "Optical Spectrum vs Wavelength"=→"Optical Spectrum vs Wavelength":cluster{"Intensity":dbl[], "Wavelength":dbl[]}, "Optical Spectrum vs Raman Shift"=→"Optical Spectrum vs Raman Shift":cluster{"Intensity":dbl[], "Raman Shift":dbl[]})
